vi "Pick&Place_ladder.vi"() -> ()   [LabVIEW 2016]
uses:
  Classes/Controllers/I-O/Copy of NI-DAQ Folder/NI-DAQ.lvclass
  D:/INTT/V1/Classes/Controllers/I-O/Copy of I-O Folder/I-O.lvclass
  Classes/Controllers/Dispenser/Copy of Ultimus V2 Folder/Ultimus V2.lvclass
  <vilib>/Analysis/coordinate.llb/2D Cartesian Coordinate Rotation (Scalar).vi
  <vilib>/Utility/file.llb/Read Delimited Spreadsheet (DBL).vi
  <vilib>/Utility/file.llb/Write Delimited Spreadsheet (DBL).vi
  Classes/Controllers/Motion/Copy of Motion Folder/Motion.lvclass
  Classes/Controllers/Camera/Copy of Controller Folder/Controller.lvclass
  <vilib>/Analysis/NI_AALPro.lvlib
  Classes/Controllers/I-O/Copy of I-O Folder/I-O.lvclass
panel:
  in  "check height?":bool
  in  "Uttimus presssure":i64=10
  out "Status":bool
  out "measured HDI top-left position":dbl[][](array[numeric])
  in  "HDI vacuum channel":i32=18
  in  "vacuum":bool=TRUE
  in  "HDI vacuum":bool
  out "measured stave size":dbl[](array[numeric])
  out "Stave mark":dbl[][](array[numeric])
  out "Center of module on stave":dbl[](array[numeric])
  out "Center of HDI from alignment mark":dbl[](array[numeric])
  out "Measured HDI size":dbl[][](array[numeric])
  out "module position on stave":dbl[][](array[numeric])
  in  "Default Stave dimension":dbl[](array[numeric])=[34.0, 472.0, -0.335295, -0.000320234]
  in  "Default Stave upper left mark":dbl[](array[numeric])=[584.376, 675.576, 70.9882, 0.000840064]
  out "Needle parking position":dbl[](array[numeric])
  in  "chip placement height\ncompensation":dbl=-0.41 format="%#_13g"
  in  "Uppler / Lower Stave":bool=TRUE
  out "Gantry current position":dbl[](array[numeric])
  in  "READ Position":bool
  in  "Needle Height Compenstation\n(glue gap)":dbl=0.33
  in  "Needle Alignment":bool
  in  "Parking position":dbl[](array[numeric])=[625.0, 625.0, 0.0, 0.01]
  in  "GOTO":bool
  in  "Default Pickup Tool Position":dbl[][](array[numeric])=[[152.226, 682.729, 36.8129, -0.0151898], [700.0, 800.0, 20.0, 0.01]]
  in  "Number of module \nto be assembled":i32=1
  in  "Default HDI alignment \nmark position":dbl[](array[numeric])=[448.322, 976.582, 74.9872, 0.000191129]
  in  "Default HDI size":dbl[](array[numeric])=[24.2437, 231.446, -0.099339, 0.000191129]
  out "# of tasks excuted":i32
  out "module on tray position":dbl[][](array[numeric])
  out "PickupTool \nCenterPosition":dbl[](array[numeric])
  in  "Inititalize":bool
  in  "Pick and place":bool
  in  "Deposit Glue":bool
  in  "Measure Pickup Tools":bool
  in  "Align Stave":bool
  out "default module position on stave":dbl[][](array[numeric])
  in  "Stop":bool
  in  "Measure HDI":bool
  # "Ladder Assembly"
  # "Sensor 0.32 -> 200 micron glue thickness\nChips 0.37-> 140 micron glue thickness"
  # "Lower\nmodule"
  # "Upper\nmodule"
  # "Chips : -0.41 -> 70 micron height gap\nSensors (feet stops the lowering)"
  # "ACTIONS"
  # "Stave infomation"
  # "Module infomation"
  # "Pick and Place"
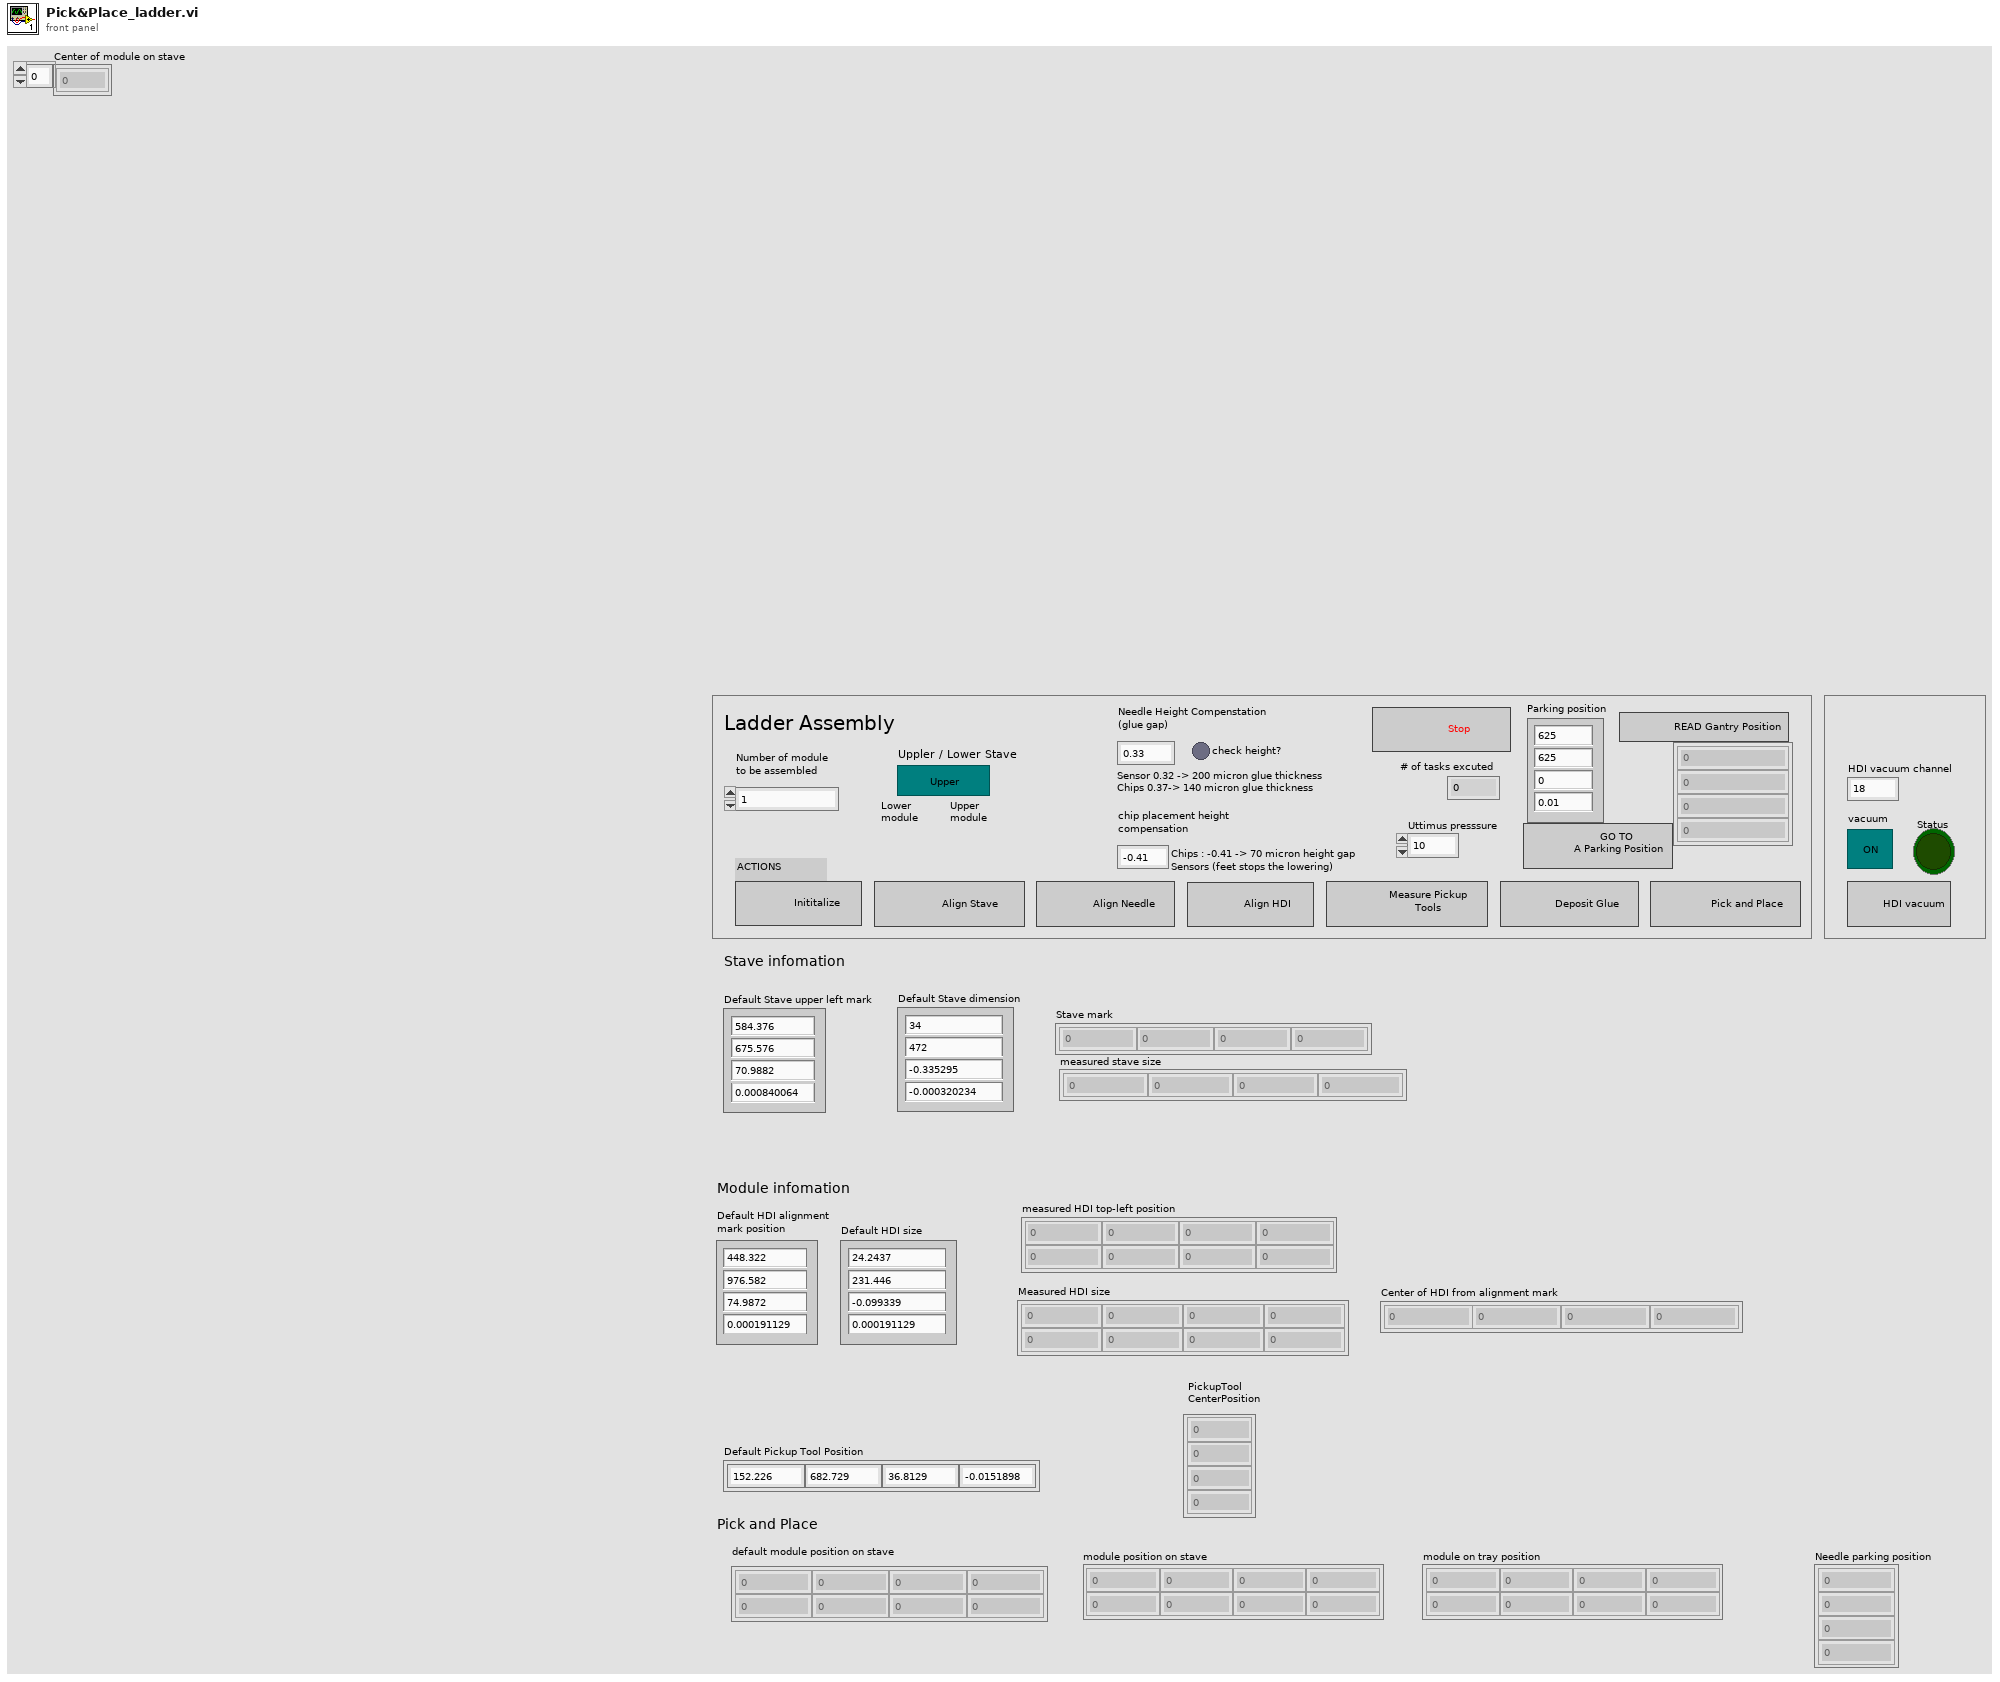
[diagram p1: front panel]
types:
  T1 = typedef "Controller.lvclass/Controllers.ctl" = cluster{"Copy of Motion.lvclass":refnum<class "Motion.lvclass">, "Copy of I-O.lvclass":refnum<class "I-O.lvclass">, "Copy of Dispenser.lvclass":refnum<class "Dispenser.lvclass">}
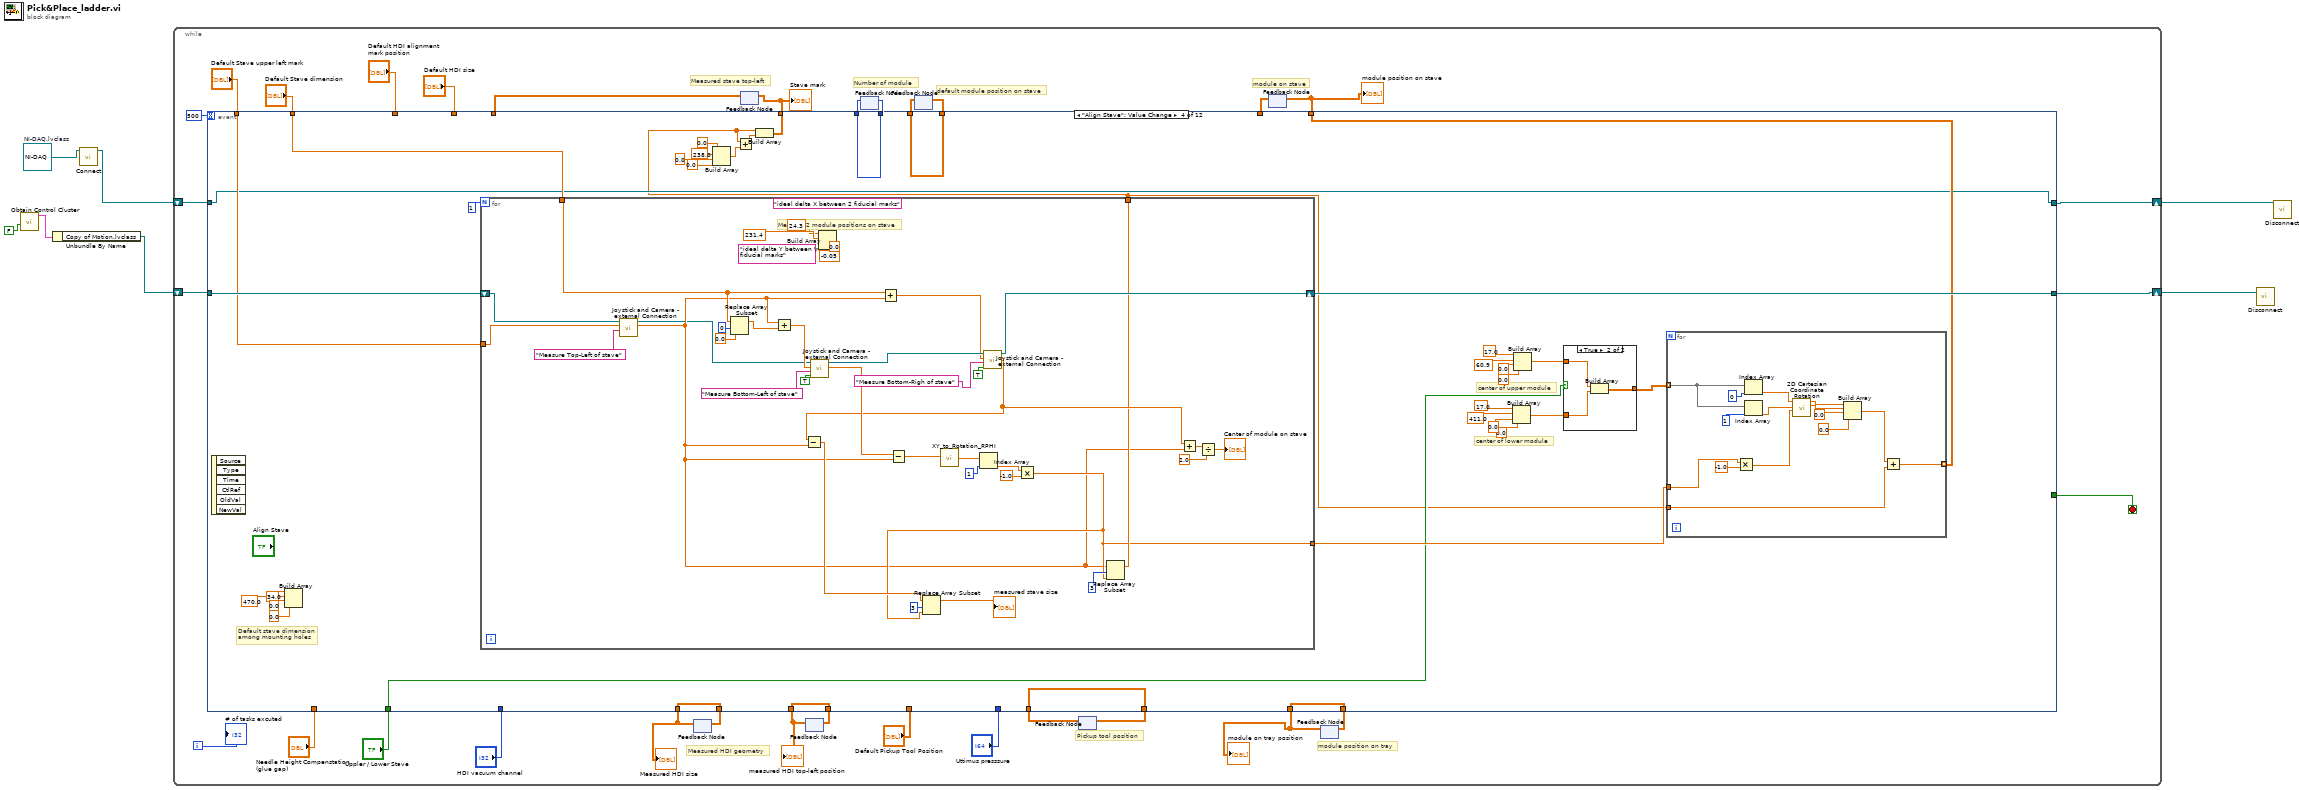
[diagram p0: block diagram]
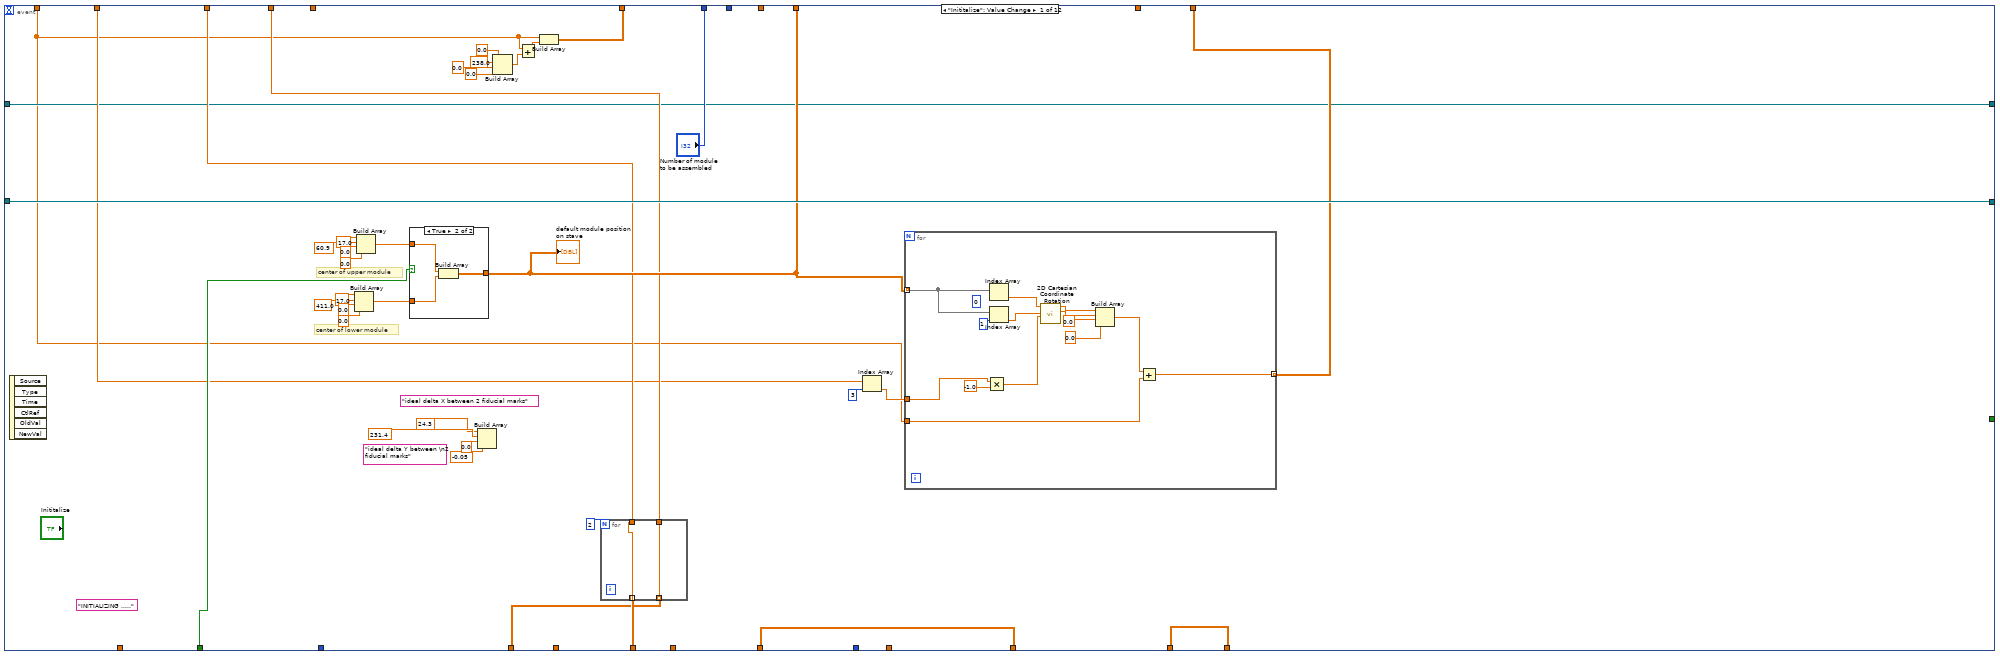
[diagram p2: hidden frame]
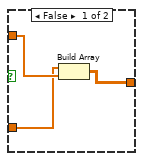
[diagram p3: hidden frame]
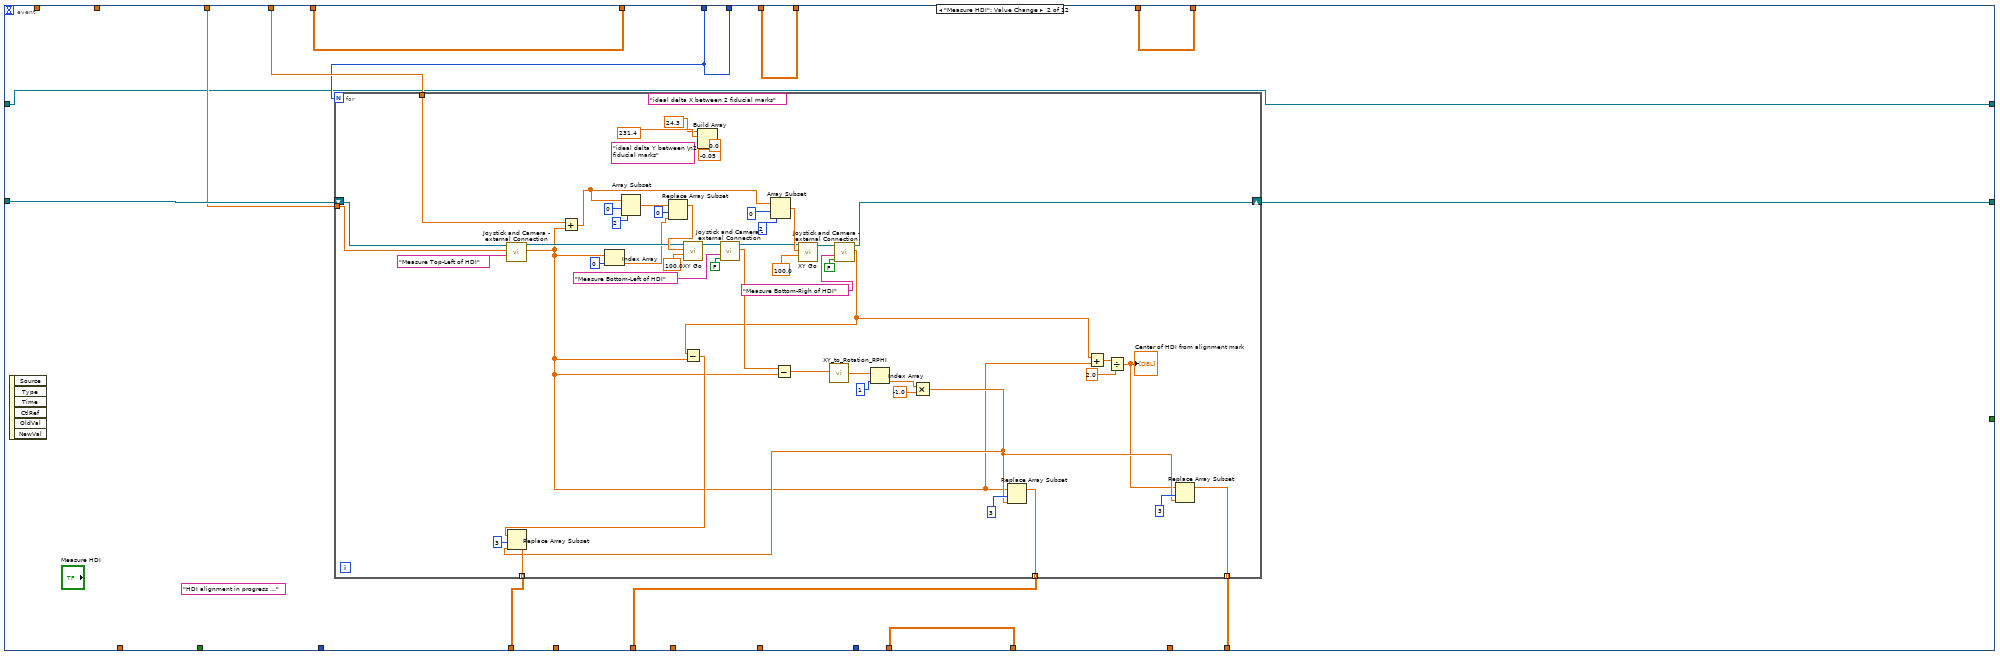
[diagram p4: hidden frame]
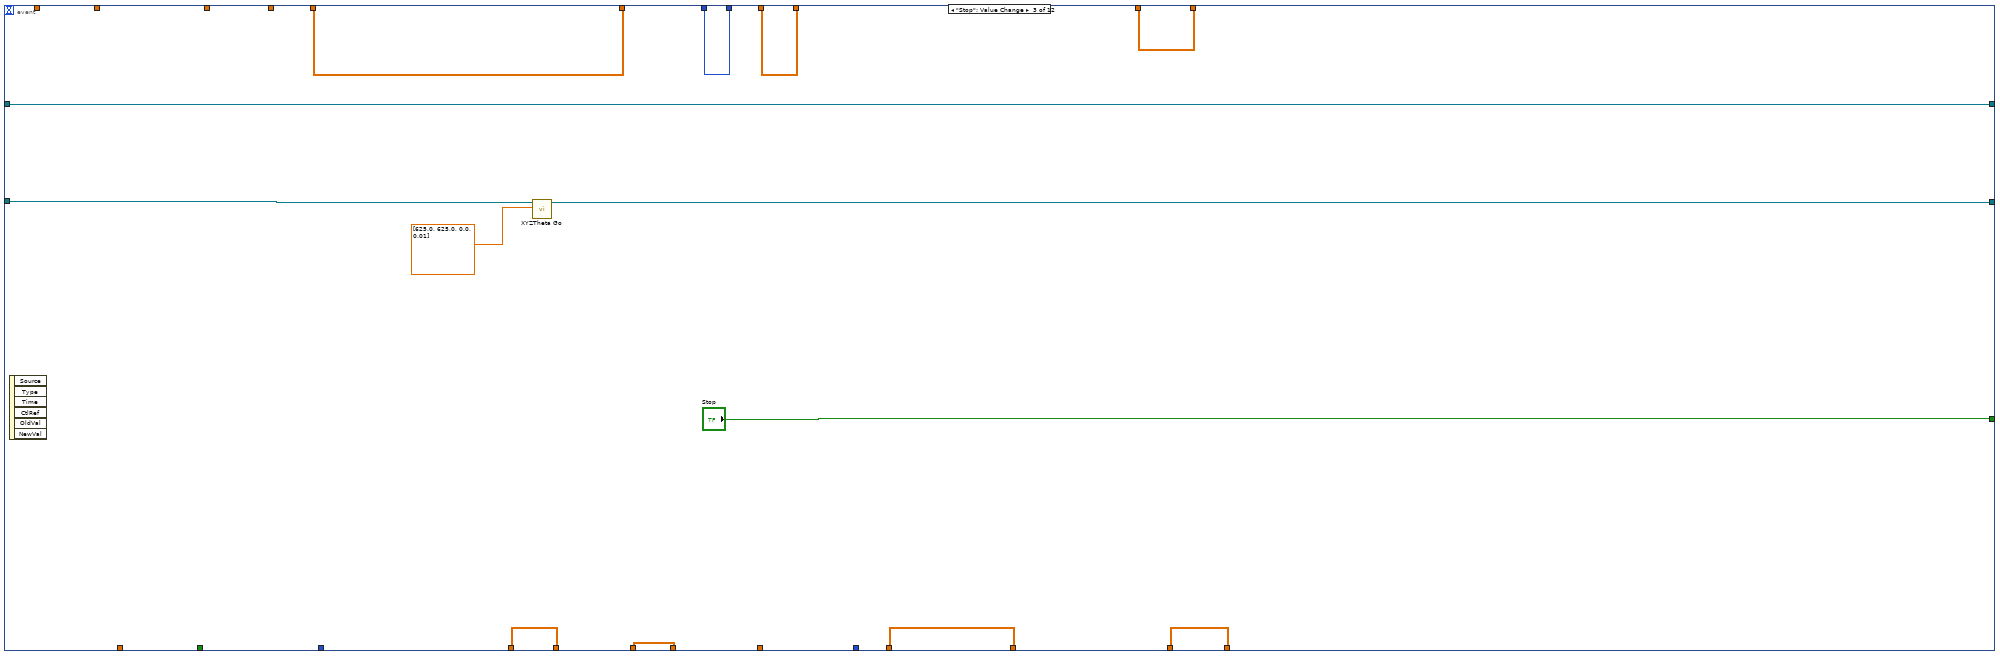
[diagram p5: hidden frame]
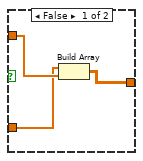
[diagram p6: hidden frame]
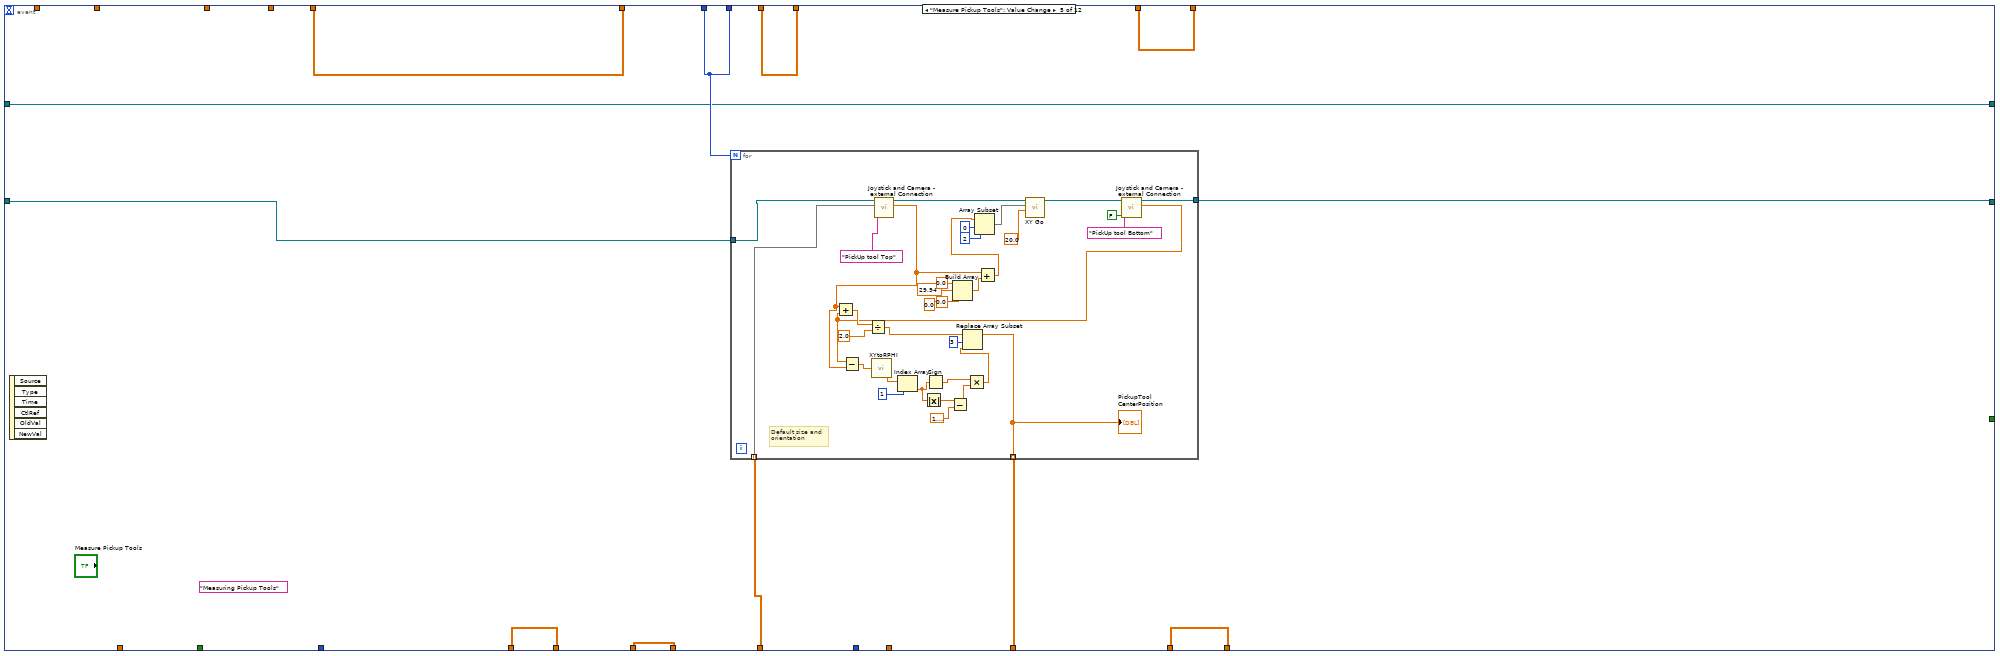
[diagram p7: hidden frame]
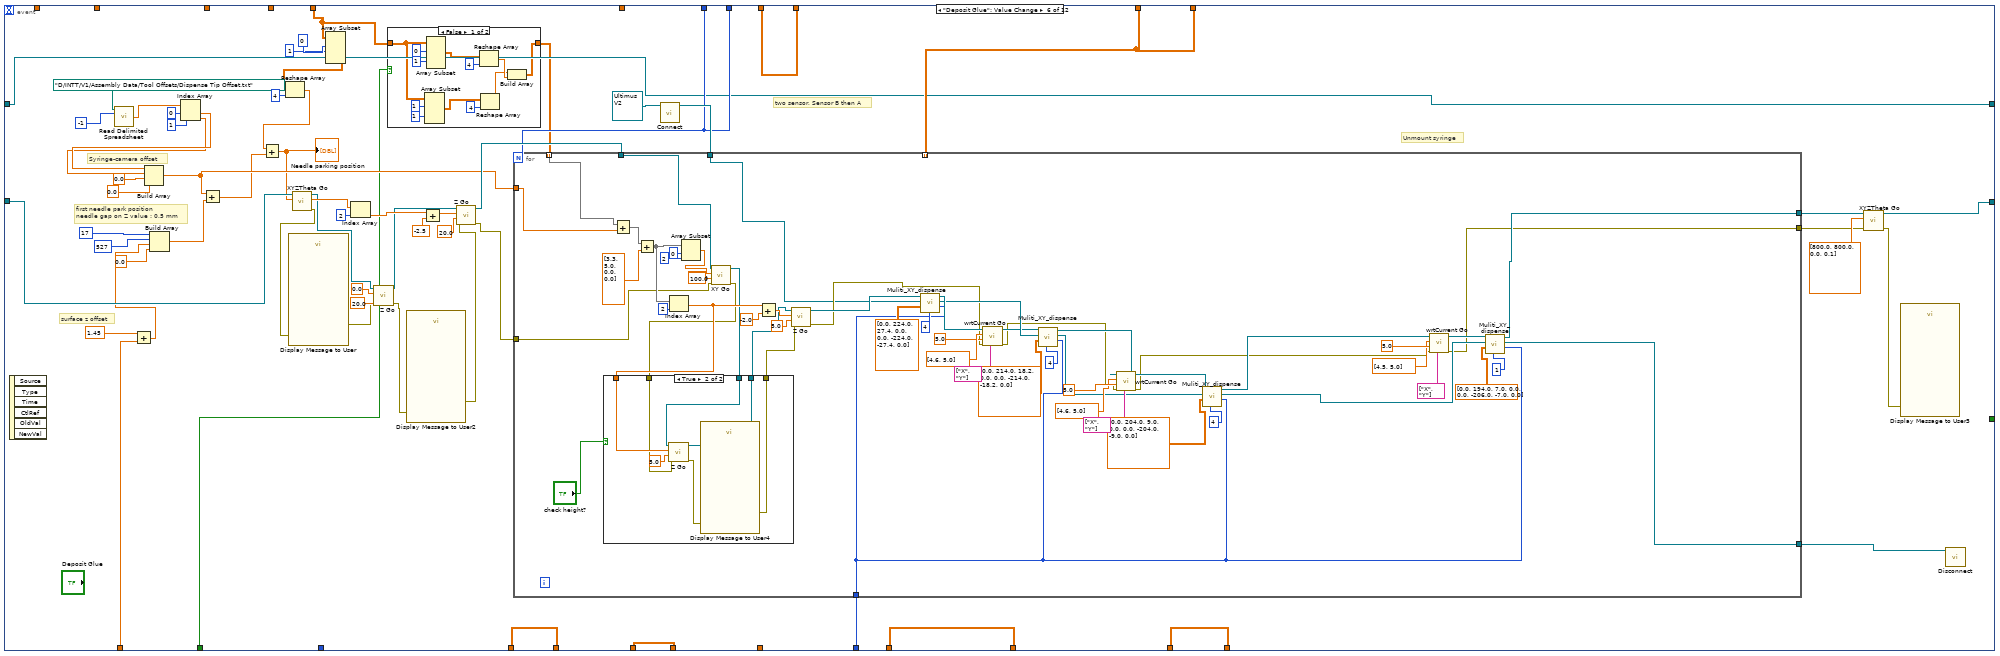
[diagram p8: hidden frame]
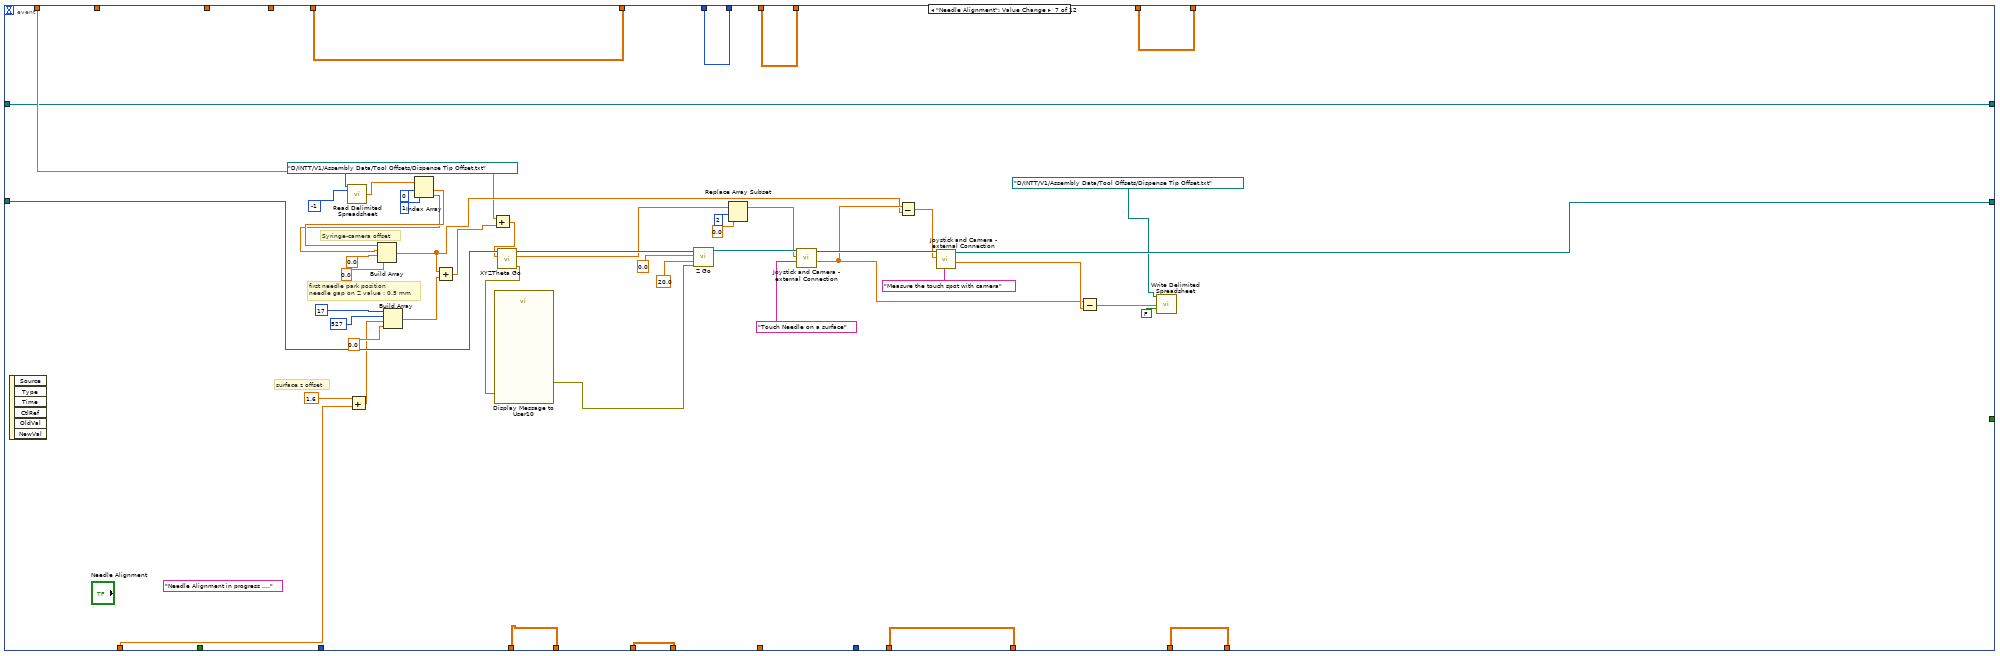
[diagram p11: hidden frame]
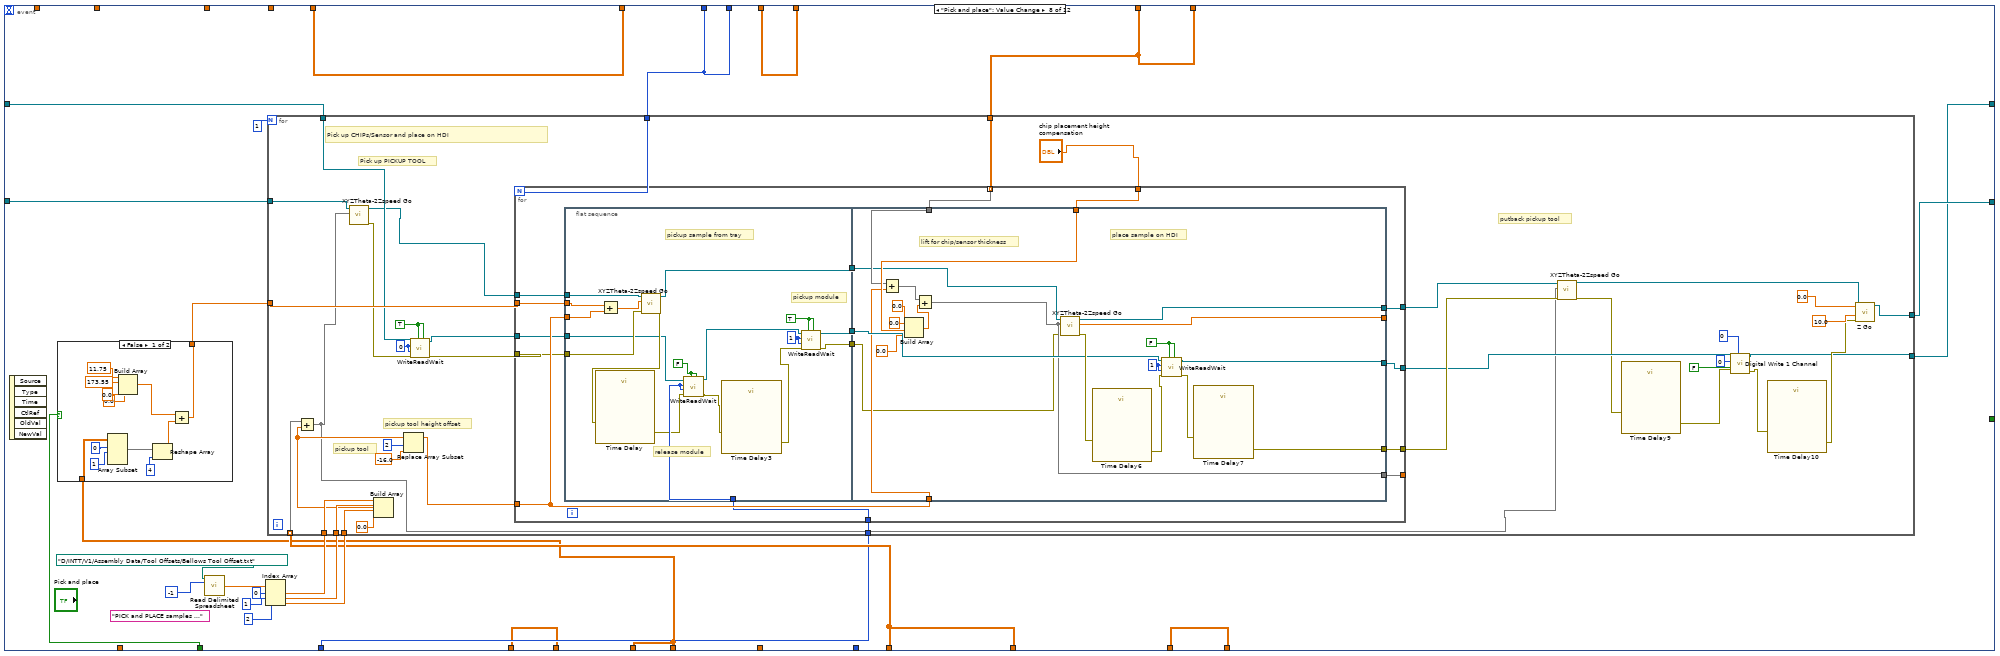
[diagram p12: hidden frame]
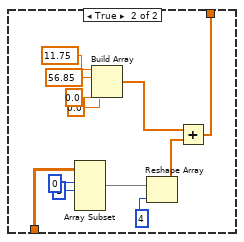
[diagram p13: hidden frame]
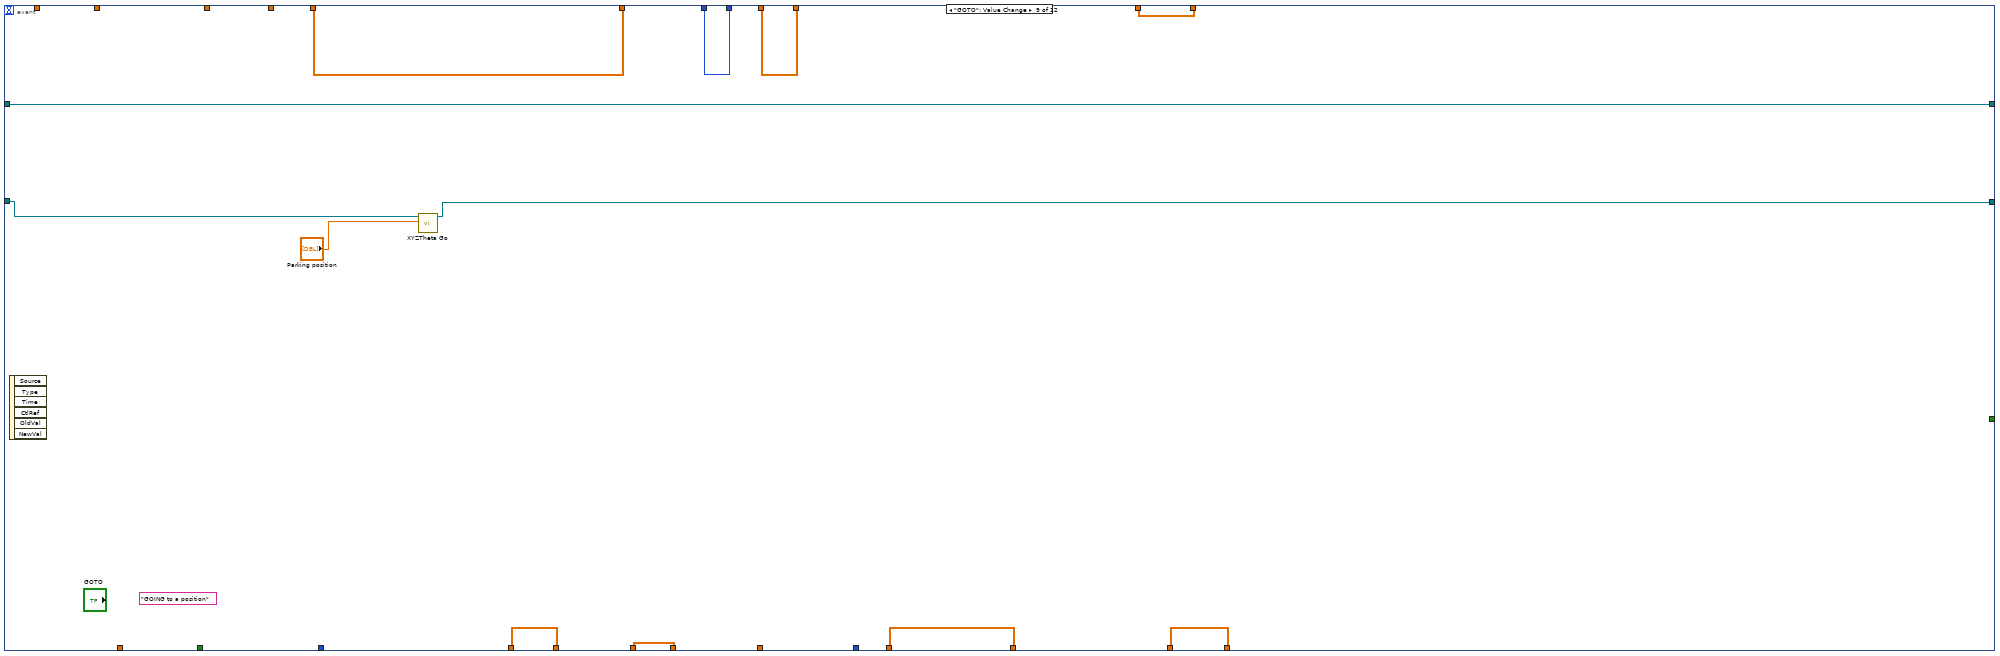
[diagram p14: hidden frame]
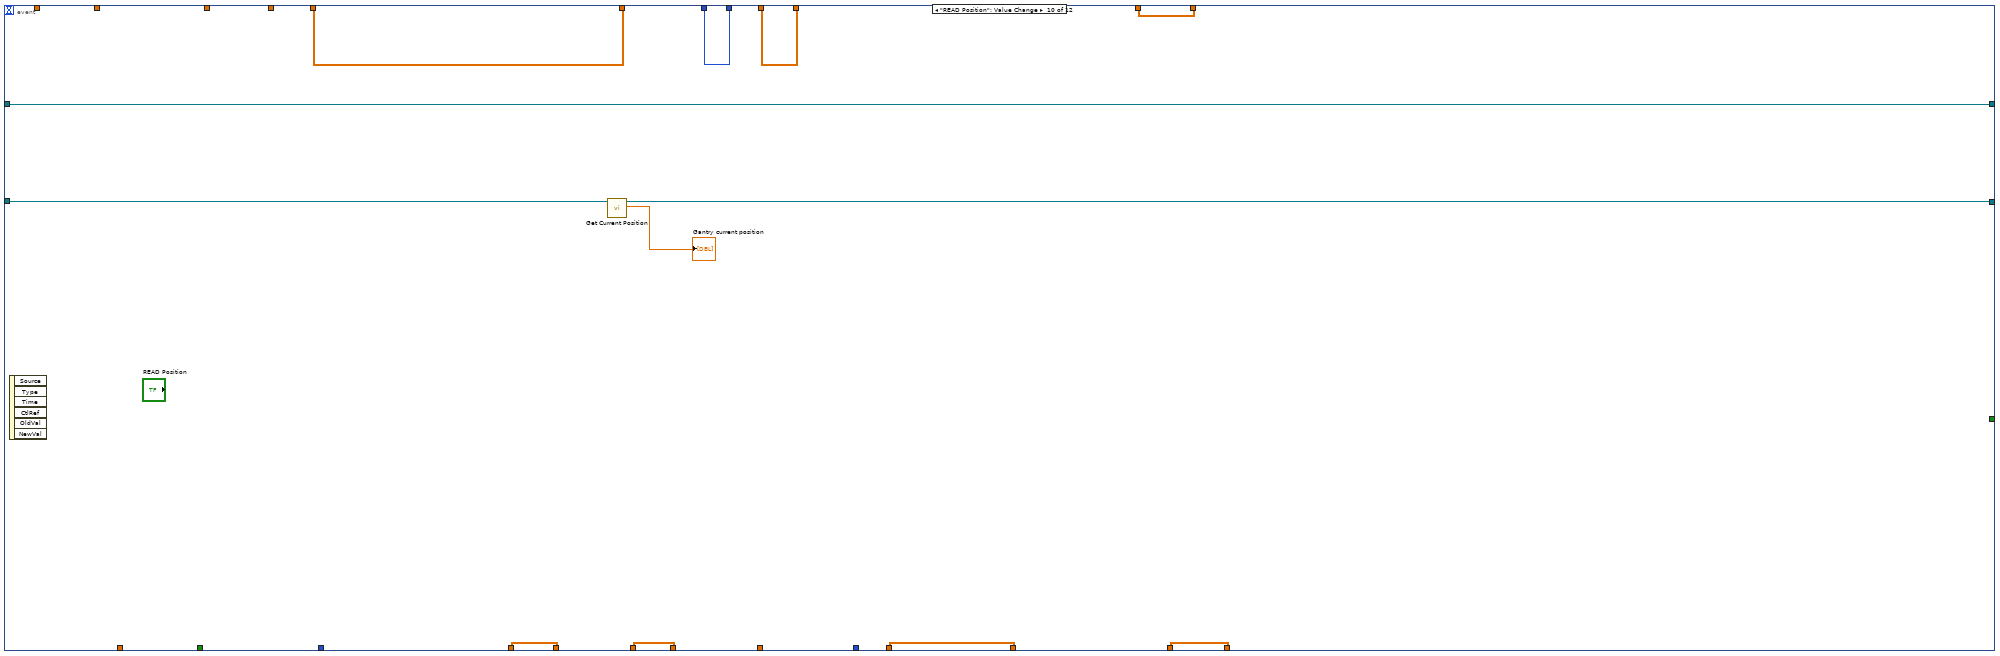
[diagram p15: hidden frame]
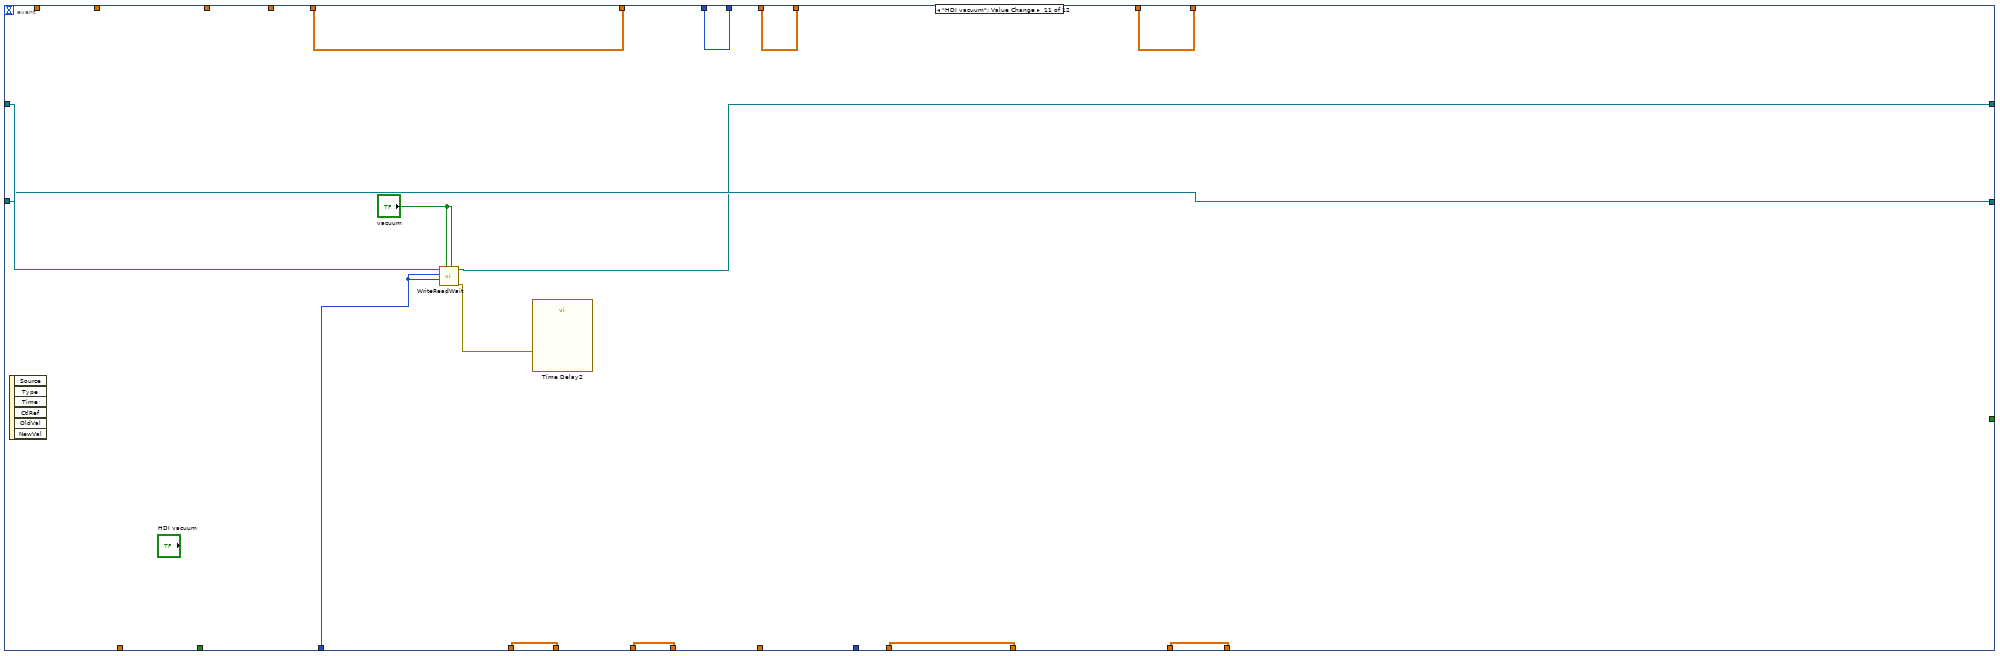
[diagram p16: hidden frame]
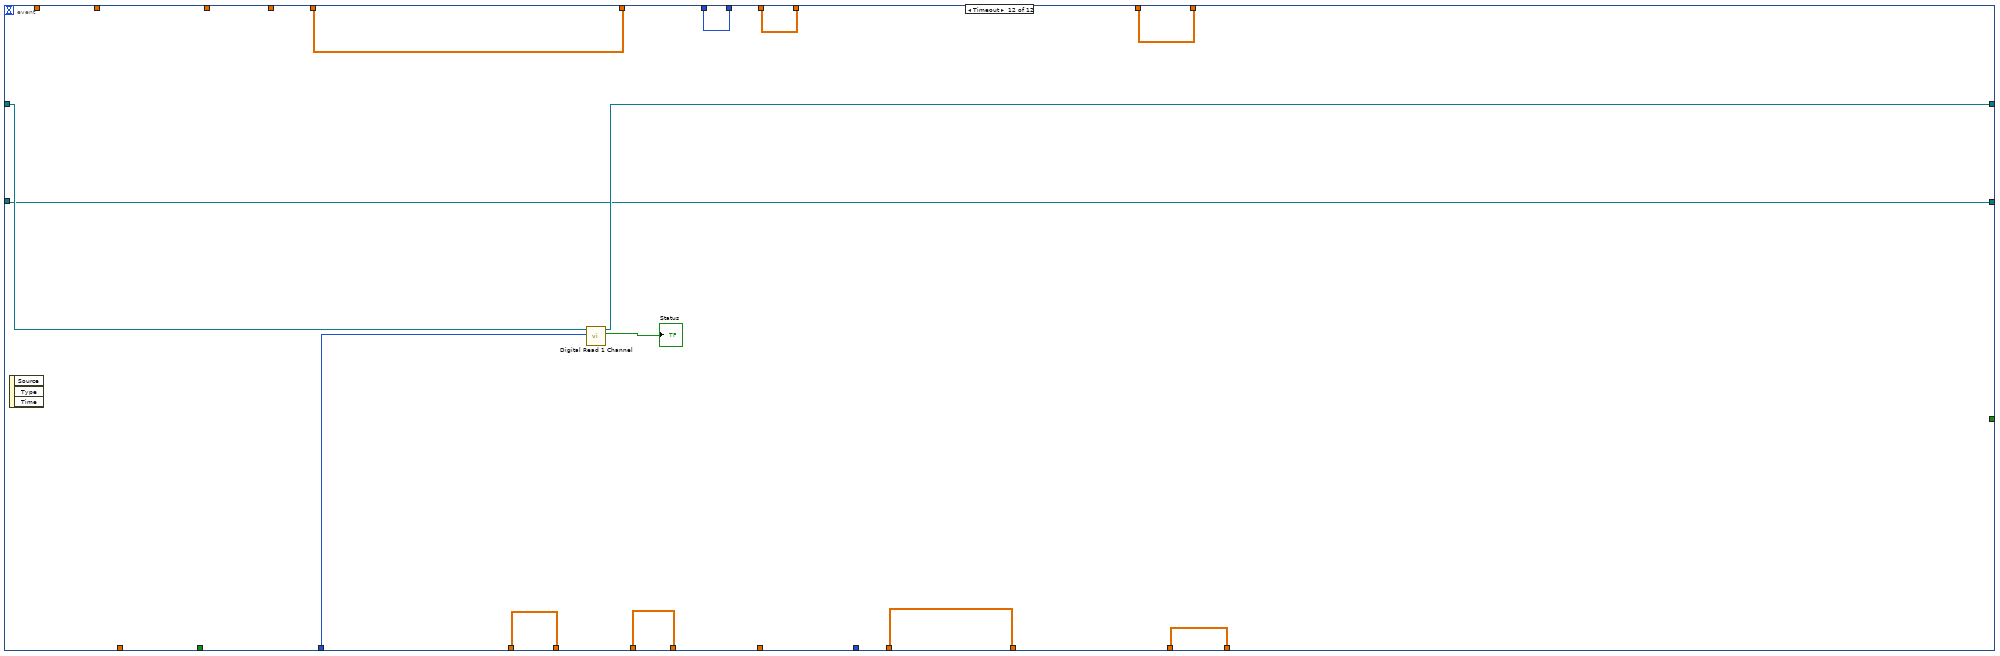
[diagram p17: hidden frame]
diagram:
  w3 = refnum<class "NI-DAQ.lvclass"> refnum  # NI-DAQ.lvclass
  n1 = call "Obtain Control Cluster.vi"("I/O"=FALSE) -> ("Control Out"=w7:T1)  [unwired: 10 in]
  n2 = Unbundle By Name(w7) -> ("Copy of Motion.lvclass"=w5:refnum<class "Motion.lvclass">)
  n3 = call-dynamic "Connect.vi"("NI-DAQ in"=w3) -> ("NI-DAQ out"=w2:refnum<class "NI-DAQ.lvclass">)  [unwired: 9 in, 1 out]
  n4 = while {
    shift-right: [w32] -> w4
    shift-left: w5 -> [w39]
    shift-right: [w11] -> w1
    shift-left: w2 -> [w15]
    i -> [w31]
    stop <- w38 stop-if-true
    # "default module position on stave"
    # "Pickup tool position"
    # "Number of module"
    # "Measured HDI geometry"
    # "module position on tray"
    # "Measured stave top-left"
    # "module on stave"
    n5 = feedback #1() -> (w36:dbl[][])  [unwired: 1 in]
    n6 = feedback #2() -> (w37:dbl[][])  [unwired: 1 in]
    n7 = feedback #3() -> (w12:dbl[][])  [unwired: 1 in]
    n8 = feedback #4() -> (w30:i32)  [unwired: 1 in]
    n9 = feedback #5() -> (w25:dbl[][])  [unwired: 1 in]
    n10 = feedback #6() -> (w33:dbl[][])  [unwired: 1 in]
    n11 = feedback #7() -> (w19:dbl[][])  [unwired: 1 in]
    n12 = feedback #8() -> (w23:dbl[][])  [unwired: 1 in]
    "module on tray position" <- w23
    n13 = event shown="[3] \"Align Stave\": Value Change" {
      selector: _ -> [_ _ _ _ _ _ _ _ _ _ _ _]
      dyn-events: _ -> [_ _ _ _ _ _ _ _ _ _ _ _]
      timeout: 500 -> [_ _ _ _ _ _ _ _ _ _ _ _]
      tunnel: w39 -> [w73 w112 w174 w204 w282 w353 w484 w530 w652 w670 w672 w693]
      tunnel: [_ _ "Stop" _ _ _ _ _ _ _ _ _] -> w38
      tunnel: [w40 w106 w169 w175 w277 _ w464 w508 w658 w666 w680 w692] -> w16
      tunnel: w37 -> [_ w106 w169 _ w277 w318 w464 w508 w658 w666 w680 w692]
      tunnel: [w50 w104 w168 w200 w276 w339 w487 w511 w655 w665 w674 w690] -> w17
      tunnel: w36 -> [_ _ w168 w200 w276 w339 w487 w511 w655 w665 w674 w690]
      tunnel: w30 -> [_ w102 w171 w205 w273 w342 w489 w515 w657 w667 w678 w685]
      tunnel: [w55 w103 w166 w207 w275 w341 w485 w518 w653 w663 w676 w687] -> w35
      tunnel: w23 -> [w55 _ w166 w207 w275 w341 w485 w518 w653 w663 w676 w687]
      tunnel: [w71 w107 w167 w212 w281 w340 w486 w519 w654 w664 w675 w688] -> w34
      tunnel: w33 -> [_ w107 w167 w212 _ w340 w486 w519 w654 w664 w675 w688]
      tunnel: [w73 w111 w172 w201 w280 w343 w476 w520 w650 w669 w672 w693] -> w32
      tunnel: ["Number of module \nto be assembled" w102 w171 w205 w273 w342 w489 w515 w657 w667 w678 w685] -> w29
      tunnel: "Default HDI alignment \nmark position" -> [w53 w110 _ _ _ _ _ _ _ _ _ _]
      tunnel: "Default HDI size" -> [w52 w109 _ _ _ _ _ _ _ _ _ _]
      tunnel: [w60 w108 w170 w206 w278 w338 w488 w517 w656 w668 w679 w691] -> w26
      tunnel: w25 -> [_ w108 w170 w206 w278 w338 w488 w517 w656 w668 w679 w691]
      tunnel: "Default Pickup Tool Position" -> [w71 _ _ _ w279 _ _ _ _ _ _ _]
      tunnel: "Uppler / Lower Stave" -> [w56 _ _ w185 _ w319 _ w506 _ _ _ _]
      tunnel: "Default Stave upper left mark" -> [w41 _ _ w203 _ _ w463 _ _ _ _ _]
      tunnel: "Default Stave dimension" -> [w49 _ _ w202 _ _ _ _ _ _ _ _]
      tunnel: [w57 w105 w164 w184 w274 w335 w465 w507 w648 w660 w677 w686] -> w18
      tunnel: w19 -> [_ w105 w164 _ w274 w335 w465 w507 w648 w660 w677 w686]
      tunnel: w15 -> [w48 w100 w162 w183 w271 w329 w461 w514 w647 w659 w684 w696]
      tunnel: [w48 w100 w162 w183 w271 w329 w461 w513 w647 w659 w671 w694] -> w11
      tunnel: "HDI vacuum channel" -> [_ _ _ _ _ _ _ w512 _ _ w681 w695]
      tunnel: [w51 w101 w163 w199 w272 w330 w462 w510 w649 w661 w673 w689] -> w13
      tunnel: w12 -> [_ _ w163 w199 w272 w330 w462 w510 w649 w661 w673 w689]
      tunnel: "Needle Height Compenstation\n(glue gap)" -> [_ _ _ _ _ w321 w457 _ _ _ _ _]
      tunnel: "Uttimus presssure" -> [_ _ _ _ _ w320 _ _ _ _ _ _]
      event "Inititalize": Value Change {
        (unwired) "INITIALIZING ....." ("String")
        (unwired) "ideal delta Y between \n2 fiducial marks"
        (unwired) "ideal delta X between 2 fiducial marks"
        # "center of lower module"
        # "center of upper module"
        n14 = event-data() -> ()  [unwired: 1 in, 6 out]
        n15 = Build Array(17.0 ("element"), 411.0 ("element"), 0.0 ("element"), 0.0 ("element")) -> (w61:dbl[])
        n16 = Build Array(17.0 ("element"), 60.9 ("element"), 0.0 ("element"), 0.0 ("element")) -> (w62:dbl[])
        n17 = case shown="True" w56 {
          tunnel: w62 -> [w82 w85]
          tunnel: w61 -> [w81 w84]
          tunnel: [w80 w83] -> w60
          frame False {
            n18 = Build Array(w81, w82) -> (w80:dbl[][])
          }
          frame True {
            n19 = Build Array(w85, w84) -> (w83:dbl[][])
          }
        }
        "default module position on stave" <- w60
        n20 = Build Array(24.3 ("y"), 231.4 ("y"), 0.0 ("element"), -0.05 ("element")) -> ()  [unwired: 1 out]
        n21 = Build Array(0.0 ("element"), 238.0 ("element"), 0.0 ("element"), 0.0 ("element")) -> (w43:dbl[])
        n22 = Add(x=w41, y=w43) -> (x+y=w42:dbl[])
        n23 = Build Array(w41, w42) -> (w40:dbl[][])
        n24 = for {
          N: 2 -> [_]
          tunnel: w53 -> [w79]
          tunnel: [w79] -> w51 mode=indexing
          tunnel: w52 -> [w78]
          tunnel: [w78] -> w50 mode=indexing
        }
        n25 = Index Array(array=w49, index=3) -> (element=w58:dbl)
        n26 = for {
          tunnel: w60 -> [w93] mode=indexing
          tunnel: w58 -> [w87]
          tunnel: w41 -> [w92]
          tunnel: [w90] -> w57 mode=indexing
          (unwired) 0 ("index")
          n27 = Multiply(x=w87, y=-1.0) -> (x*y=w88:dbl)
          n28 = Index Array(array=w93) -> (element=w96:dbl)  [unwired: 1 in]
          n29 = Index Array(array=w93, index=1) -> (element=w95:dbl)
          n30 = call-poly <vilib>:"2D Cartesian Coordinate Rotation.vi"("theta"=w88, "y"=w95, "x"=w96) -> ("y out"=w98:dbl, "x out"=w97:dbl)  [unwired: 6 in, 1 out]
          n31 = Build Array(w97, w98, 0.0 ("element"), 0.0 ("element")) -> (w91:dbl[])
          n32 = Add(x=w91, y=w92) -> (x+y=w90:dbl[])
        }
      }
      event "Measure HDI": Value Change {
        (unwired) "HDI alignment in progress ..." ("String")
        n33 = event-data() -> ()  [unwired: 1 in, 6 out]
        n34 = for {
          N: w102 -> [_]
          tunnel: w109 -> [w124]
          shift-right: [w121] -> w111
          shift-left: w112 -> [w122]
          tunnel: w110 -> [w123]
          tunnel: [w158] -> w101 mode=indexing
          tunnel: [w157] -> w104 mode=indexing
          tunnel: [w114] -> w103 mode=indexing
          (unwired) "ideal delta Y between \n2 fiducial marks"
          (unwired) "ideal delta X between 2 fiducial marks"
          n35 = call "Joystick and Camera - external Connection.vi"("Motion in"=w122, "XYZTheta"=w123, "Measurement Point"="Measure Top-Left of HDI") -> ("Motion out"=w137:refnum<class "Motion.lvclass">, "Sum"=w113:dbl[])  [unwired: 4 in, 2 out]
          n36 = Add(x=w124, y=w113) -> (x+y=w141:dbl[])
          n37 = Index Array(array=w113, index=0) -> (element=w128:dbl)
          n38 = Array Subset(array=w141, index=0, length=2) -> (w140:dbl[])
          n39 = Replace Array Subset(array=w140, new element=w128, index=0) -> (w138:dbl[])
          n40 = call-dynamic "XY Go.vi"("Speed"=100.0, "XY"=w138, "Motion in"=w137) -> ("Motion out"=w145:refnum<class "Motion.lvclass">)  [unwired: 7 in, 1 out]
          n41 = Build Array(24.3 ("y"), 231.4 ("y"), 0.0 ("element"), -0.05 ("element")) -> ()  [unwired: 1 out]
          n42 = call "Joystick and Camera - external Connection.vi"("Motion in"=w145, "Measurement Point"="Measure Bottom-Left of HDI", "Inital GO"=FALSE) -> ("Motion out"=w136:refnum<class "Motion.lvclass">, "Sum"=w127:dbl[])  [unwired: 4 in, 2 out]
          n43 = Array Subset(array=w141, index=0, length=2) -> (w151:dbl[])
          n44 = Subtract(x=w127, y=w113) -> (x-y=w135:dbl[])
          n45 = call-dynamic "XY Go.vi"("Speed"=100.0, "XY"=w151, "Motion in"=w136) -> ("Motion out"=w155:refnum<class "Motion.lvclass">)  [unwired: 7 in, 1 out]
          n46 = call "XY_to_Rotation_RPHI.vi"("X-Y"=w135) -> ("r-phi"=w131:dbl[])
          n47 = call "Joystick and Camera - external Connection.vi"("Motion in"=w155, "Measurement Point"="Measure Bottom-Righ of HDI", "Inital GO"=FALSE) -> ("Motion out"=w121:refnum<class "Motion.lvclass">, "Sum"=w118:dbl[])  [unwired: 4 in, 2 out]
          n48 = Subtract(x=w118, y=w113) -> (x-y=w119:dbl[])
          n49 = Index Array(array=w131, index=1) -> (element=w125:dbl)
          n50 = Multiply(x=w125, y=-1.0) -> (x*y=w116:dbl)
          n51 = Replace Array Subset(array=w119, new element=w116, index=3) -> (w157:dbl[])
          n52 = Replace Array Subset(array=w113, new element=w116, index=3) -> (w158:dbl[])
          n53 = Add(x=w118, y=w113) -> (x+y=w160:dbl[])
          n54 = Divide(x=w160, y=2.0) -> (x/y=w115:dbl[])
          "Center of HDI from alignment mark" <- w115
          n55 = Replace Array Subset(array=w115, new element=w116, index=3) -> (w114:dbl[])
        }
      }
      event "Stop": Value Change {
        n56 = event-data() -> ()  [unwired: 1 in, 6 out]
        n57 = call "XYZTheta Go.vi"("XYZTheta In"=dbl[] [625.0, 625.0, 0.0, 0.01], "Motion in"=w174) -> ("Motion out"=w172:refnum<class "Motion.lvclass">)  [unwired: 7 in, 2 out]
      }
      event "Align Stave": Value Change {
        # "center of lower module"
        # "center of upper module"
        # "Default stave dimension\namong mounting holes"
        # "Measure 2 module positions on stave"
        n58 = event-data() -> ()  [unwired: 1 in, 6 out]
        n59 = Build Array(34.0 ("element"), 470.0 ("element"), 0.0 ("element"), 0.0 ("element")) -> ()  [unwired: 1 out]
        n60 = for {
          N: 1 -> [_]
          tunnel: w202 -> [w240]
          shift-right: [w250] -> w201
          shift-left: w204 -> [w251]
          tunnel: w203 -> [w252]
          tunnel: [w245] -> w177
          tunnel: [w243] -> w187
          (unwired) "ideal delta Y between \n2 fiducial marks"
          (unwired) "ideal delta X between 2 fiducial marks"
          n61 = call "Joystick and Camera - external Connection.vi"("Motion in"=w251, "XYZTheta"=w252, "Measurement Point"="Measure Top-Left of stave") -> ("Motion out"=w234:refnum<class "Motion.lvclass">, "Sum"=w236:dbl[])  [unwired: 4 in, 2 out]
          n62 = Replace Array Subset(array=w240, new element=0.0 ("new element/subarray"), index=0) -> (w237:dbl[])
          n63 = Add(x=w236, y=w237) -> (x+y=w235:dbl[])
          n64 = call "Joystick and Camera - external Connection.vi"("Motion in"=w234, "XYZTheta"=w235, "Measurement Point"="Measure Bottom-Left of stave", "Inital GO"=TRUE) -> ("Motion out"=w242:refnum<class "Motion.lvclass">, "Sum"=w255:dbl[])  [unwired: 3 in, 2 out]
          n65 = Build Array(24.3 ("y"), 231.4 ("y"), 0.0 ("element"), -0.05 ("element")) -> ()  [unwired: 1 out]
          n66 = Add(x=w240, y=w236) -> (x+y=w241:dbl[])
          n67 = Subtract(x=w255, y=w236) -> (x-y=w261:dbl[])
          n68 = call "XY_to_Rotation_RPHI.vi"("X-Y"=w261) -> ("r-phi"=w257:dbl[])
          n69 = Index Array(array=w257, index=1) -> (element=w253:dbl)
          n70 = call "Joystick and Camera - external Connection.vi"("Motion in"=w242, "XYZTheta"=w241, "Measurement Point"="Measure Bottom-Righ of stave", "Inital GO"=TRUE) -> ("Motion out"=w250:refnum<class "Motion.lvclass">, "Sum"=w247:dbl[])  [unwired: 3 in, 2 out]
          n71 = Subtract(x=w247, y=w236) -> (x-y=w248:dbl[])
          n72 = Multiply(x=w253, y=-1.0) -> (x*y=w243:dbl)
          n73 = Replace Array Subset(array=w248, new element=w243, index=3) -> (→"measured stave size":dbl[])
          n74 = Replace Array Subset(array=w236, new element=w243, index=3) -> (w245:dbl[])
          n75 = Add(x=w247, y=w236) -> (x+y=w269:dbl[])
          n76 = Divide(x=w269, y=2.0) -> (x/y=→"Center of module on stave":dbl[])
        }
        n77 = Build Array(0.0 ("element"), 238.0 ("element"), 0.0 ("element"), 0.0 ("element")) -> (w178:dbl[])
        n78 = Add(x=w177, y=w178) -> (x+y=w176:dbl[])
        n79 = Build Array(w177, w176) -> (w175:dbl[][])
        n80 = Build Array(17.0 ("element"), 411.0 ("element"), 0.0 ("element"), 0.0 ("element")) -> (w189:dbl[])
        n81 = Build Array(17.0 ("element"), 60.9 ("element"), 0.0 ("element"), 0.0 ("element")) -> (w190:dbl[])
        n82 = case shown="True" w185 {
          tunnel: w190 -> [w230 w233]
          tunnel: w189 -> [w229 w232]
          tunnel: [w228 w231] -> w188
          frame False {
            n83 = Build Array(w229, w230) -> (w228:dbl[][])
          }
          frame True {
            n84 = Build Array(w233, w232) -> (w231:dbl[][])
          }
        }
        n85 = for {
          tunnel: w188 -> [w221] mode=indexing
          tunnel: w187 -> [w216]
          tunnel: w177 -> [w220]
          tunnel: [w218] -> w184 mode=indexing
          n86 = Multiply(x=w216, y=-1.0) -> (x*y=w215:dbl)
          n87 = Index Array(array=w221, index=0) -> (element=w224:dbl)
          n88 = Index Array(array=w221, index=1) -> (element=w223:dbl)
          n89 = call-poly <vilib>:"2D Cartesian Coordinate Rotation.vi"("theta"=w215, "y"=w223, "x"=w224) -> ("y out"=w226:dbl, "x out"=w225:dbl)  [unwired: 6 in, 1 out]
          n90 = Build Array(w225, w226, 0.0 ("element"), 0.0 ("element")) -> (w219:dbl[])
          n91 = Add(x=w219, y=w220) -> (x+y=w218:dbl[])
        }
      }
      event "Measure Pickup Tools": Value Change {
        (unwired) "Measuring Pickup Tools" ("String")
        n92 = event-data() -> ()  [unwired: 1 in, 6 out]
        n93 = for {
          N: w273 -> [_]
          tunnel: [w306] -> w281 mode=indexing
          tunnel: w282 -> [w310]
          tunnel: [w292] -> w280
          tunnel: w279 -> [w291] mode=indexing
          # "Default size and\norientation"
          n94 = call "Joystick and Camera - external Connection.vi"("Motion in"=w310, "XYZTheta"=w291, "Measurement Point"="PickUp tool Top") -> ("Motion out"=w286:refnum<class "Motion.lvclass">, "Sum"=w309:dbl[])  [unwired: 4 in, 2 out]
          n95 = Build Array(0.0 ("element"), 29.94 ("element"), 0.0 ("element"), 0.0 ("element")) -> (w297:dbl[])
          n96 = Add(x=w309, y=w297) -> (x+y=w283:dbl[])
          n97 = Array Subset(array=w283, index=0, length=2) -> (w284:dbl[])
          n98 = call-dynamic "XY Go.vi"("Speed"=20.0, "XY"=w284, "Motion in"=w286) -> ("Motion out"=w285:refnum<class "Motion.lvclass">)  [unwired: 7 in, 1 out]
          n99 = call "Joystick and Camera - external Connection.vi"("Motion in"=w285, "Measurement Point"="PickUp tool Bottom", "Inital GO"=FALSE) -> ("Motion out"=w292:refnum<class "Motion.lvclass">, "Sum"=w308:dbl[])  [unwired: 4 in, 2 out]
          n100 = Add(x=w309, y=w308) -> (x+y=w315:dbl[])
          n101 = Subtract(x=w308, y=w309) -> (x-y=w307:dbl[])
          n102 = Divide(x=w315, y=2.0) -> (x/y=w312:dbl[])
          n103 = call "XYtoRPHI.vi"("X-Y"=w307) -> ("r-phi"=w313:dbl[])
          n104 = Index Array(array=w313, index=1) -> (element=w301:dbl)
          n105 = Absolute Value(x=w301) -> (abs(x)=w304:dbl)
          n106 = Sign(1:w301) -> (0:w302:dbl)
          n107 = Subtract(x=w304, y=1.5707963267948966) -> (x-y=w303:dbl)
          n108 = Multiply(x=w302, y=w303) -> (x*y=w300:dbl)
          n109 = Replace Array Subset(array=w312, new element=w300, index=3) -> (w306:dbl[])
          "PickupTool \nCenterPosition" <- w306
        }
      }
      event "Deposit Glue": Value Change {
        # "surface z offset"
        # "two sensor, Sensor B then A"
        # "Unmount syringe"
        # "first needle park position\nneedle gap on Z value : 0.5 mm"
        # "Syringe-camera offset"
        n110 = event-data() -> ()  [unwired: 1 in, 6 out]
        n111 = call-poly <vilib>:"Read Delimited Spreadsheet.vi"("file path (dialog if empty)"=path "D:/INTT/V1/Assembly Data/Tool Offsets/Dispense Tip Offset.txt", "number of rows (all:-1)"=-1) -> ("first row"=w373:dbl[])  [unwired: 8 in, 5 out]
        n112 = Add(x=1.45 ("element"), y=w321) -> (x+y=w333:dbl)
        n113 = Build Array(17, 527, w333, 0.0 ("element")) -> (w366:dbl[])
        n114 = Index Array(array=w373, index #1=0 ("index"), index #2=1 ("index")) -> (element #1=w368:dbl, element #2=w365:dbl)
        n115 = Build Array(w368, w365, 0.0 ("element"), 0.0 ("element")) -> (w348:dbl[])
        n116 = Add(x=w348, y=w366) -> (x+y=w337:dbl[])
        n117 = Array Subset(array=w318, index (row)=0, length (row)=1 ("length")) -> (w325:dbl[][])  [unwired: 2 in]
        n118 = Reshape Array(w325, 4 ("dimension size")) -> (w324:dbl[])
        n119 = Add(x=w324, y=w337) -> (x+y=w336:dbl[])
        "Needle parking position" <- w336
        n120 = call "XYZTheta Go.vi"("XYZTheta In"=w336, "Motion in"=w353) -> ("error out"=w364:errorcluster, "XYZTheta Out"=w362:dbl[], "Motion out"=w352:refnum<class "Motion.lvclass">)  [unwired: 7 in]
        n121 = call "Display Message to User"("error in (no error)"=w364) -> ("error out"=w354:errorcluster)  [unwired: 9 in, 1 out]
        n122 = Index Array(array=w362, index=2) -> (element=w358:dbl)
        n123 = call-dynamic "Z Go.vi"("error in (no error)"=w354, "Speed"=20.0, "Position"=0.0, "Motion in"=w352) -> ("error out"=w351:errorcluster, "Motion out"=w357:refnum<class "Motion.lvclass">)  [unwired: 6 in]
        n124 = case shown="False" w319 {
          tunnel: w318 -> [w381 w390]
          tunnel: [w378 w390] -> w317
          frame False {
            n125 = Array Subset(array=w381, index (row)=1 ("index"), length (row)=1 ("length")) -> (w382:dbl[][])  [unwired: 2 in]
            n126 = Array Subset(array=w381, index (row)=0 ("index"), length (row)=1 ("length")) -> (w385:dbl[][])  [unwired: 2 in]
            n127 = Reshape Array(w385, 4 ("dimension size")) -> (w380:dbl[])
            n128 = Reshape Array(w382, 4 ("dimension size")) -> (w379:dbl[])
            n129 = Build Array(w379, w380) -> (w378:dbl[][])
          }
          frame True {
          }
        }
        n130 = call "Display Message to User2"("error in (no error)"=w351) -> ("error out"=w350:errorcluster)  [unwired: 9 in, 1 out]
        n131 = Add(x=w358, y=-2.5) -> (x+y=w359:dbl)
        n132 = call-dynamic "Z Go.vi"("error in (no error)"=w350, "Speed"=20.0, "Position"=w359, "Motion in"=w357) -> ("error out"=w323:errorcluster, "Motion out"=w349:refnum<class "Motion.lvclass">)  [unwired: 6 in]
        n133 = call-dynamic "Connect.vi"("Ultimus V in"=refnum<class "Ultimus V2.lvclass"> refnum ("Ultimus V2.lvclass")) -> ("Ultimus V out"=w347:refnum<class "Ultimus V2.lvclass">)  [unwired: 9 in, 1 out]
        n134 = for {
          N: w342 -> [_]
          tunnel: w349 -> [w405]
          tunnel: w347 -> [w404]
          tunnel: w348 -> [w406]
          tunnel: w335 -> [_] mode=indexing
          tunnel: w317 -> [w407] mode=indexing
          tunnel: [w403] -> w332
          tunnel: [w402] -> w331
          tunnel: w323 -> [w398]
          tunnel: [w399] -> w322
          tunnel: w320 -> [w397]
          (unwired) 100.0 ("Speed")
          n135 = Add(x=w407, y=w406) -> (x+y=w437:dbl[])
          n136 = Add(x=w437, y=dbl[] [3.3, 5.0, 0.0, 0.0]) -> (x+y=w438:dbl[])
          n137 = Index Array(array=w438, index=2) -> (element=w395:dbl)
          n138 = Array Subset(array=w438, index=0, length=2) -> (w413:dbl[])
          n139 = call-dynamic "XY Go.vi"("error in (no error)"=w398, "Speed"=100.0, "XY"=w413, "Motion in"=w405) -> ("error out"=w393:errorcluster, "Motion out"=w394:refnum<class "Motion.lvclass">)  [unwired: 6 in]
          n140 = case shown="True" "check height?" {
            tunnel: w395 -> [_ w454]
            tunnel: w394 -> [w447 w453]
            tunnel: w393 -> [w448 w452]
            tunnel: [w448 w450] -> w392
            tunnel: [w447 w449] -> w391
            frame False {
            }
            frame True {
              n141 = call-dynamic "Z Go.vi"("error in (no error)"=w452, "Speed"=5.0, "Position"=w454, "Motion in"=w453) -> ("error out"=w451:errorcluster, "Motion out"=w449:refnum<class "Motion.lvclass">)  [unwired: 6 in]
              n142 = call "Display Message to User4"("error in (no error)"=w451) -> ("error out"=w450:errorcluster)  [unwired: 9 in, 1 out]
            }
          }
          n143 = Add(x=w395, y=-2.0) -> (x+y=w412:dbl)
          n144 = call-dynamic "Z Go.vi"("error in (no error)"=w392, "Speed"=5.0, "Position"=w412, "Motion in"=w391) -> ("error out"=w410:errorcluster, "Motion out"=w411:refnum<class "Motion.lvclass">)  [unwired: 6 in]
          n145 = call "Muliti_XY_dispense.vi"("Pressure"=w397, "Path count"=4, "distances"=dbl[][] [[0.0, 224.0], [27.4, 0.0], [0.0, -224.0], [-27.4, 0.0]], "Ultimus V in"=w404, "Motion in"=w411) -> ("Ultimus V out"=w431:refnum<class "Ultimus V2.lvclass">, "Motion out"=w436:refnum<class "Motion.lvclass">)  [unwired: 5 in]
          n146 = call-dynamic "wrtCurrent Go.vi"("axis names"=string[] ["X", "Y"], "error in (no error)"=w410, "Speed"=5.0, "distances"=dbl[] [4.6, 5.0], "Motion in"=w436) -> ("error out"=w401:errorcluster, "Motion out"=w430:refnum<class "Motion.lvclass">)  [unwired: 5 in]
          n147 = call "Muliti_XY_dispense.vi"("Pressure"=w397, "Path count"=4, "distances"=dbl[][] [[0.0, 214.0], [18.2, 0.0], [0.0, -214.0], [-18.2, 0.0]], "Ultimus V in"=w431, "Motion in"=w430) -> ("Ultimus V out"=w423:refnum<class "Ultimus V2.lvclass">, "Motion out"=w422:refnum<class "Motion.lvclass">)  [unwired: 5 in]
          n148 = call-dynamic "wrtCurrent Go.vi"("axis names"=string[] ["X", "Y"], "error in (no error)"=w401, "Speed"=5.0, "distances"=dbl[] [4.6, 5.0], "Motion in"=w422) -> ("error out"=w400:errorcluster, "Motion out"=w421:refnum<class "Motion.lvclass">)  [unwired: 5 in]
          n149 = call "Muliti_XY_dispense.vi"("Pressure"=w397, "Path count"=4, "distances"=dbl[][] [[0.0, 204.0], [9.0, 0.0], [0.0, -204.0], [-9.0, 0.0]], "Ultimus V in"=w423, "Motion in"=w421) -> ("Ultimus V out"=w408:refnum<class "Ultimus V2.lvclass">, "Motion out"=w409:refnum<class "Motion.lvclass">)  [unwired: 5 in]
          n150 = call-dynamic "wrtCurrent Go.vi"("axis names"=string[] ["X", "Y"], "error in (no error)"=w400, "Speed"=5.0, "distances"=dbl[] [4.5, 5.0], "Motion in"=w409) -> ("error out"=w399:errorcluster, "Motion out"=w415:refnum<class "Motion.lvclass">)  [unwired: 5 in]
          n151 = call "Muliti_XY_dispense.vi"("Pressure"=w397, "Path count"=1, "distances"=dbl[][] [[0.0, 194.0], [7.0, 0.0], [0.0, -206.0], [-7.0, 0.0]], "Ultimus V in"=w408, "Motion in"=w415) -> ("Ultimus V out"=w402:refnum<class "Ultimus V2.lvclass">, "Motion out"=w403:refnum<class "Motion.lvclass">)  [unwired: 5 in]
        }
        n152 = call "XYZTheta Go.vi"("error in (no error)"=w322, "XYZTheta In"=dbl[] [800.0, 800.0, 0.0, 0.1], "Motion in"=w332) -> ("error out"=w345:errorcluster, "Motion out"=w343:refnum<class "Motion.lvclass">)  [unwired: 6 in, 1 out]
        n153 = call "Display Message to User3"("error in (no error)"=w345) -> ()  [unwired: 9 in, 2 out]
        n154 = call-dynamic "Disconnect.vi"("Ultimus V in"=w331) -> ()  [unwired: 9 in, 1 out]
      }
      event "Needle Alignment": Value Change {
        (unwired) "Needle Alignment in progress ...." ("String")
        # "surface z offset"
        # "first needle park position\nneedle gap on Z value : 0.5 mm"
        # "Syringe-camera offset"
        n155 = event-data() -> ()  [unwired: 1 in, 6 out]
        n156 = call-poly <vilib>:"Read Delimited Spreadsheet.vi"("file path (dialog if empty)"=path "D:/INTT/V1/Assembly Data/Tool Offsets/Dispense Tip Offset.txt", "number of rows (all:-1)"=-1) -> ("first row"=w502:dbl[])  [unwired: 8 in, 5 out]
        n157 = Add(x=1.6 ("element"), y=w457) -> (x+y=w456:dbl)
        n158 = Build Array(17, 527, w456, 0.0 ("element")) -> (w495:dbl[])
        n159 = Index Array(array=w502, index #1=0 ("index"), index #2=1 ("index")) -> (element #1=w497:dbl, element #2=w494:dbl)
        n160 = Build Array(w497, w494, 0.0 ("element"), 0.0 ("element")) -> (w469:dbl[])
        n161 = Add(x=w469, y=w495) -> (x+y=w467:dbl[])
        n162 = Add(x=w463, y=w467) -> (x+y=w466:dbl[])
        n163 = call "XYZTheta Go.vi"("XYZTheta In"=w466, "Motion in"=w484) -> ("error out"=w493:errorcluster, "XYZTheta Out"=w474:dbl[], "Motion out"=w483:refnum<class "Motion.lvclass">)  [unwired: 7 in]
        n164 = call "Display Message to User10"("error in (no error)"=w493) -> ("error out"=w490:errorcluster)  [unwired: 9 in, 1 out]
        n165 = call-dynamic "Z Go.vi"("error in (no error)"=w490, "Speed"=20.0, "Position"=0.0, "Motion in"=w483) -> ("Motion out"=w482:refnum<class "Motion.lvclass">)  [unwired: 6 in, 1 out]
        n166 = Replace Array Subset(array=w474, new element=0.0 ("new element/subarray"), index=2) -> (w471:dbl[])
        n167 = call "Joystick and Camera - external Connection.vi"("Motion in"=w482, "XYZTheta"=w471, "Measurement Point"="Touch Needle on a surface") -> ("Motion out"=w480:refnum<class "Motion.lvclass">, "Gantry"=w470:dbl[])  [unwired: 4 in, 2 out]
        n168 = Subtract(x=w470, y=w469) -> (x-y=w468:dbl[])
        n169 = call "Joystick and Camera - external Connection.vi"("Motion in"=w480, "XYZTheta"=w468, "Measurement Point"="Measure the touch spot with camera") -> ("Motion out"=w476:refnum<class "Motion.lvclass">, "Gantry"=w479:dbl[])  [unwired: 4 in, 2 out]
        n170 = Subtract(x=w470, y=w479) -> (x-y=w478:dbl[])
        n171 = call-poly <vilib>:"Write Delimited Spreadsheet.vi"("file path (dialog if empty)"=path "D:/INTT/V1/Assembly Data/Tool Offsets/Dispense Tip Offset.txt", "1D data"=w478, "append to file? (new file:F)"=FALSE) -> ()  [unwired: 11 in, 2 out]
      }
      event "Pick and place": Value Change {
        (unwired) "PICK and PLACE samples ..." ("String")
        n172 = event-data() -> ()  [unwired: 1 in, 6 out]
        n173 = case shown="False" w506 {
          tunnel: w510 -> [w532 w554]
          tunnel: [w531 w553] -> w509
          frame False {
            n174 = Array Subset(array=w532, index (row)=0 ("index"), length (row)=1 ("length")) -> (w534:dbl[][])  [unwired: 2 in]
            n175 = Build Array(11.75 ("element"), 173.55 ("element"), 0.0 ("element"), 0.0 ("element")) -> (w538:dbl[])
            n176 = Reshape Array(w534, 4 ("dimension size")) -> (w533:dbl[])
            n177 = Add(x=w538, y=w533) -> (x+y=w531:dbl[])
          }
          frame True {
            n178 = Array Subset(array=w554, index (row)=0 ("index"), length (row)=1 ("length")) -> (w544:dbl[][])  [unwired: 2 in]
            n179 = Build Array(11.75 ("element"), 56.85 ("element"), 0.0 ("element"), 0.0 ("element")) -> (w548:dbl[])
            n180 = Reshape Array(w544, 4 ("dimension size")) -> (w543:dbl[])
            n181 = Add(x=w548, y=w543) -> (x+y=w553:dbl[])
          }
        }
        n182 = call-poly <vilib>:"Read Delimited Spreadsheet.vi"("file path (dialog if empty)"=path "D:/INTT/V1/Assembly Data/Tool Offsets/Bellows Tool Offset.txt", "number of rows (all:-1)"=-1) -> ("first row"=w527:dbl[])  [unwired: 8 in, 5 out]
        n183 = Index Array(array=w527, index #1=0 ("index"), index #2=1 ("index"), index #3=2 ("index")) -> (element #1=w523:dbl, element #2=w522:dbl, element #3=w521:dbl)
        n184 = for {
          N: 1 -> [_]
          tunnel: w530 -> [w560]
          tunnel: [w583] -> w520
          tunnel: w519 -> [w592] mode=indexing
          tunnel: [w569] -> w513
          tunnel: w514 -> [w559]
          tunnel: w523 -> [w585]
          tunnel: w522 -> [w584]
          tunnel: w521 -> [w582]
          tunnel: w515 -> [w576]
          tunnel: w512 -> [w562]
          tunnel: w509 -> [w561]
          tunnel: w507 -> [w557]
          w571 = 0 ("Write")
          w574 = TRUE ("Write Value")
          # "putback pickup tool"
          # "pickup tool"
          # "pickup tool height offset"
          # "Pick up PICKUP TOOL"
          # "Pick up CHIPs/Sensor and place on HDI"
          n185 = Build Array(w585, w584, w582, 0.0 ("element")) -> (w581:dbl[])
          n186 = Add(x=w592, y=w581) -> (x+y=w555:dbl[])
          n187 = call "XYZTheta-2Zspeed Go.vi"("XYZTheta In"=w555, "Motion in"=w560) -> ("error out"=w558:errorcluster, "Motion out"=w556:refnum<class "Motion.lvclass">)  [unwired: 7 in, 1 out]
          n188 = Replace Array Subset(array=w581, new element=-16.0 ("t"), index=2) -> (w579:dbl[])
          n189 = call "WriteReadWait.vi"("Read Value"=w574, "Write Value"=w574, "error in (no error)"=w558, "Read"=w571, "Write"=w571, "I-O in"=w559) -> ("error out"=w573:errorcluster, "I-O out"=w572:refnum<class "NI-DAQ.lvclass">)  [unwired: 4 in]
          n190 = for {
            N: w576 -> [_]
            tunnel: w556 -> [w606]
            tunnel: w579 -> [w605]
            tunnel: w573 -> [w604]
            tunnel: [w603] -> w586
            tunnel: w572 -> [w602]
            tunnel: [w601] -> w570
            tunnel: [w600] -> w578
            tunnel: "chip placement height\ncompensation" -> [w599]
            tunnel: w562 -> [w596]
            tunnel: w561 -> [w595]
            tunnel: w557 -> [w594] mode=indexing
            tunnel: [w593] -> _
            n191 = flat-sequence {
              tunnel: [w625] -> w607
              tunnel: w606 -> [w624]
              tunnel: w605 -> [w623]
              tunnel: w604 -> [w621]
              tunnel: w602 -> [w613]
              tunnel: [w620] -> w598
              tunnel: [w617] -> w597
              tunnel: w596 -> [w610]
              tunnel: w595 -> [w616]
              tunnel: w607 -> [w628]
              tunnel: [w646] -> w603
              tunnel: [w645] -> _
              tunnel: w605 -> [w631]
              tunnel: [w634] -> w601
              tunnel: [w644] -> w600
              tunnel: w599 -> [w640]
              tunnel: w598 -> [w636]
              tunnel: w597 -> [w626]
              tunnel: w594 -> [w630]
              tunnel: [w627] -> w593
              frame #0 {
                w611 = FALSE ("Write Value")
                w618 = TRUE ("Write Value")
                w619 = 1 ("Write")
                # "pickup module"
                # "release module"
                # "pickup sample from tray"
                n192 = Add(x=w616, y=w623) -> (x+y=w622:dbl[])
                n193 = call "XYZTheta-2Zspeed Go.vi"("error in (no error)"=w621, "XYZTheta In"=w622, "Motion in"=w624) -> ("error out"=w614:errorcluster, "Motion out"=w625:refnum<class "Motion.lvclass">)  [unwired: 6 in, 1 out]
                n194 = call "Time Delay"("error in (no error)"=w614) -> ("error out"=w609:errorcluster)  [unwired: 10 in]
                n195 = call "WriteReadWait.vi"("Read Value"=w611, "Write Value"=w611, "error in (no error)"=w609, "Read"=w610, "Write"=w610, "I-O in"=w613) -> ("error out"=w608:errorcluster, "I-O out"=w612:refnum<class "NI-DAQ.lvclass">)  [unwired: 4 in]
                n196 = call "Time Delay3"("error in (no error)"=w608) -> ("error out"=w615:errorcluster)  [unwired: 10 in]
                n197 = call "WriteReadWait.vi"("Read Value"=w618, "Write Value"=w618, "error in (no error)"=w615, "Read"=w619, "Write"=w619, "I-O in"=w612) -> ("error out"=w617:errorcluster, "I-O out"=w620:refnum<class "NI-DAQ.lvclass">)  [unwired: 4 in]
              }
              frame #1 {
                w635 = 1 ("Write")
                w637 = FALSE ("Write Value")
                # "lift for chip/sensor thickness"
                # "place sample on HDI"
                n198 = Add(x=w630, y=w631) -> (x+y=w641:dbl[])
                n199 = Build Array(0.0 ("element"), 0.0 ("element"), w640, 0.0 ("element")) -> (w632:dbl[])
                n200 = Add(x=w641, y=w632) -> (x+y=w627:dbl[])
                n201 = call "XYZTheta-2Zspeed Go.vi"("error in (no error)"=w626, "XYZTheta In"=w627, "Motion in"=w628) -> ("error out"=w639:errorcluster, "XYZTheta Out"=w645:dbl[], "Motion out"=w646:refnum<class "Motion.lvclass">)  [unwired: 6 in]
                n202 = call "Time Delay6"("error in (no error)"=w639) -> ("error out"=w638:errorcluster)  [unwired: 10 in]
                n203 = call "WriteReadWait.vi"("Read Value"=w637, "Write Value"=w637, "error in (no error)"=w638, "Read"=w635, "Write"=w635, "I-O in"=w636) -> ("error out"=w633:errorcluster, "I-O out"=w634:refnum<class "NI-DAQ.lvclass">)  [unwired: 4 in]
                n204 = call "Time Delay7"("error in (no error)"=w633) -> ("error out"=w644:errorcluster)  [unwired: 10 in]
              }
            }
          }
          n205 = call "XYZTheta-2Zspeed Go.vi"("error in (no error)"=w578, "XYZTheta In"=w555, "Motion in"=w586) -> ("error out"=w565:errorcluster, "Motion out"=w590:refnum<class "Motion.lvclass">)  [unwired: 6 in, 1 out]
          n206 = call "Time Delay9"("error in (no error)"=w565) -> ("error out"=w567:errorcluster)  [unwired: 10 in]
          n207 = call-dynamic "Digital Write 1 Channel.vi"("DAQ Module"=0, "error constant"=w567, "Value"=FALSE, "Channel"=0, "NI-DAQ.lvclass"=w570) -> ("error IO"=w566:errorcluster, "NI-DAQ.lvclass 2"=w569:refnum<class "NI-DAQ.lvclass">)  [unwired: 5 in]
          n208 = call "Time Delay10"("error in (no error)"=w566) -> ("error out"=w587:errorcluster)  [unwired: 10 in]
          n209 = call-dynamic "Z Go.vi"("error in (no error)"=w587, "Speed"=10.0, "Position"=0.0 ("new element/subarray"), "Motion in"=w590) -> ("Motion out"=w583:refnum<class "Motion.lvclass">)  [unwired: 6 in, 1 out]
        }
      }
      event "GOTO": Value Change {
        (unwired) "GOING to a position" ("String")
        n210 = event-data() -> ()  [unwired: 1 in, 6 out]
        n211 = call "XYZTheta Go.vi"("XYZTheta In"="Parking position", "Motion in"=w652) -> ("Motion out"=w650:refnum<class "Motion.lvclass">)  [unwired: 7 in, 2 out]
      }
      event "READ Position": Value Change {
        n212 = event-data() -> ()  [unwired: 1 in, 6 out]
        n213 = call-dynamic "Get Current Position.vi"("Motion in"=w670) -> ("XYZTheta Out"=→"Gantry current position":dbl[], "Motion out"=w669:refnum<class "Motion.lvclass">)  [unwired: 8 in, 1 out]
      }
      event "HDI vacuum": Value Change {
        n214 = event-data() -> ()  [unwired: 1 in, 6 out]
        n215 = call "WriteReadWait.vi"("Read Value"="vacuum", "Write Value"="vacuum", "Read"=w681, "Write"=w681, "I-O in"=w684) -> ("error out"=w682:errorcluster, "I-O out"=w671:refnum<class "NI-DAQ.lvclass">)  [unwired: 5 in]
        n216 = call "Time Delay2"("error in (no error)"=w682) -> ()  [unwired: 10 in, 1 out]
      }
      event Timeout {
        n217 = event-data() -> ()  [unwired: 1 in, 3 out]
        n218 = call-dynamic "Digital Read 1 Channel.vi"("Read"=w695, "NI-DAQ in"=w696) -> ("Value"=→"Status":bool, "NI-DAQ out"=w694:refnum<class "NI-DAQ.lvclass">)  [unwired: 7 in, 1 out]
      }
    }
    "Measured HDI size" <- w17
    "module position on stave" <- w18
    "Stave mark" <- w16
    "measured HDI top-left position" <- w13
    n219 = feedback-in #1(w17) -> ()
    n220 = feedback-in #2(w16) -> ()
    n221 = feedback-in #3(w13) -> ()
    n222 = feedback-in #4(w29) -> ()
    n223 = feedback-in #5(w26) -> ()
    n224 = feedback-in #6(w34) -> ()
    n225 = feedback-in #7(w18) -> ()
    n226 = feedback-in #8(w35) -> ()
    "# of tasks excuted" <- w31
  }
  n227 = call-dynamic "Disconnect.vi"("Controller in"=w4) -> ()  [unwired: 9 in, 1 out]
  n228 = call-dynamic "Disconnect.vi"("I-O in"=w1) -> ()  [unwired: 9 in, 1 out]
